vi "MegaAwesome_9_24_12a_JW.vi"() -> ()   [LabVIEW 2011]
uses:
  MegaAwesome_States.ctl
  <vilib>/Utility/inputDevices.llb/keyboardAcquire.vi
  <vilib>/Utility/file.llb/Read From Spreadsheet File (string).vi
  <vilib>/Utility/file.llb/Write To Spreadsheet File (string).vi
panel:
  out "Image Center X":i32
  in  "Disable Flag":bool
  out "Index":string
  out "ROI Descriptor out":T1 {"Contours"."Type" items=["No Selection", "Point", "Line", "Rectangle", "Oval", "Polygon", "Freehand Region", "Annulus", "Unused2", "Unused3", "Broken Line", "Freehand Line", "Rotated Rectangle"]}
  out "ROI Descriptor":T1 {"Contours"."Type" items=["No Selection", "Point", "Line", "Rectangle", "Oval", "Polygon", "Freehand Region", "Annulus", "Unused2", "Unused3", "Broken Line", "Freehand Line", "Rotated Rectangle"]}
  in  "Slider Min":dbl=5.0
  in  "Slider Max":dbl=5.0
  out "Opj X Axis":string
  out "X Axis Display Type":string
  in  "Index-Sat":dbl=5.0
  in  "Index-Lin":dbl=5.0
  in  "IndexLog-Lin":dbl=5.0
  in  "IndexLog-Sat":dbl=5.0 caption="Num Pts"
  out "Lin Id-Log Used":dbl[](array[numeric])
  out "Lin-Vg Array-Log Used":dbl[](array[numeric])
  in  "New: Comments":string
  out "Save Array":string[][](array[string])
  out "Folder Index":i32 caption="Length"
  out "Sat Id-Used":dbl[](array[numeric])
  out "Sat Vg Array-Used":dbl[](array[numeric])
  out "Vg Array-Log-Used":dbl[](array[numeric])
  out "Sat Id-Log-Used":dbl[](array[numeric])
  out "Lin Id-Used":dbl[](array[numeric])
  out "Lin-Vg Array-Used":dbl[](array[numeric])
  out "Lin Vd":dbl
  out "Recorded Prop":T2
  out "Current State":T3
  in  "Main Tab Control":T4(tab)
  in  "OE Link":bool
  in  "Transfer File":path
  out "Transfer Folder":path
  in  "1) Transport":bool caption="2) Transport"
  in  "Image Analysis":bool caption="1) Image Analysis"
  in  "Transport\nFolder":path caption="Transport Folder"
  out "Transport\nFile":path=path "D:/UserData/Desktop/Jeremy/WFU/Research/Programs/VI mods/Image Not Found.png" caption="Transport File"
  in  "Image Folder":path
  out "Image File":path=path "D:/UserData/Desktop/Jeremy/WFU/Research/Programs/VI mods/Image Not Found.png"
  out "Fabrication Prop":T5
  out "Distances":dbl[](array[numeric])
  in  "Zoom":i16(slide)=-3 scale=-5.0..5.0
  in  "Magnification":u16(ring) items=["5x", "10x", "20x", "50x", "80x"]
  in  "Undo Button":bool
  in  "Remove Button":bool
  in  "Transfer Plots":T6(tab)=enum."Saturation"
  in  "Lin-Trans Slider":dbl(slide) step=1.0 scale=-4.0..4.0 scale format="%#_1p"
  out "Sqrt-Lin":cluster{dbl[], dbl[]}[](graph)
  in  "Sat-Trans Slider":dbl(slide) step=1.0 scale=-4.0..4.0 scale format="%#_1p"
  out "Sqrt-Sat":cluster{dbl[], dbl[]}[](graph)
  out "Raw- Lin":cluster{dbl[], dbl[]}[](graph)
  out "Raw- Sat":cluster{dbl[], dbl[]}[](graph)
  in  "Log Plots":enum32{"Linear", "Saturation", "Transport"}(tab)=enum."Saturation"
  in  "Lin-Log Slider":dbl(slide) step=1.0 scale=-4.0..4.0 scale format="%#_1p"
  out "Lin-Log":cluster{dbl[], dbl[]}[](graph)
  in  "Sat-Log Slider":dbl(slide) step=1.0 scale=-4.0..4.0 scale format="%#_1p"
  out "Sat-Log":cluster{dbl[], dbl[]}[](graph)
  out "Transport":cluster{dbl[], dbl[]}[](graph)
  out "Transport Name:":string
  in  "Manual Controls":T7
  in  "File Controls":T8
  out "Date Recorded":string="Date Recorded" caption="Measured"
  out "Data Name:":string
  out "Image Name":string
  out "Date Created":string caption="Fabricated"
  in  "Comments:":string
  out "Rec: Length":dbl caption="Length" format="%#_3g"
  out "Rec: Width":dbl caption="Width" format="%#_4g"
  out "Rec: Dielectric (d)":dbl caption="Dielectric (d)" format="%#_3g"
  in  "New: Dielectric":dbl
  in  "New: Length":dbl
  in  "New: Width":dbl
  out "Rec: Temp":dbl caption="Sample Temp" format="%.1f"
  in  "New: Temp":dbl format="%.1f"
  out "Image Out":T9(plugin-control)
  in  "Num Pts":dbl=5.0
  in  "Num Pts Log":dbl=5.0 caption="Num Pts"
  out "Recorded Values Cluster":T10
  out "Calculated Values Cluster":T10 caption="Recorded Values Cluster"
  out "Re-Calculated Values Cluster":T10 caption="Recorded Values Cluster"
  in  "Independant Variable:":string(combo)="Length (um):"
  out "Image Preview":T9(plugin-control)
  out "Total Width":dbl
  in  "Index Array":u16(ring) caption="Index" items=["1A", "1A", "1A", "1A", "1A", "1A", "1A", "1A", "1A", "1A", "1A", "1A", "1A", "1A", "1A", "1A", "1A", "1A", "1A", "1A", "1A", "1A", "1A", "1A", "1A", "1A", "1A", "1A", "1A", "1A", "1A", "1A", "1A", "1A", "1A", "1A", "1A"]
  in  "Room Temp":dbl=294.0 caption="Room Temp (K)"
  out "No Image\n File":path=path "\\\\acad1\\physics/Jurchescu-group/JW-PD/Mega Awesome/Image Not Found.png" caption="No Image File"
  out "Origin Project File":path=path "\\\\acad1\\physics/Jurchescu-group/JW-PD/Group Library/Origin Project Files/DeviceData_8_10_12a_JW.opj"
  out "No Transport\n File":path=path "\\\\acad1\\physics/Jurchescu-group/JW-PD/Mega Awesome/No Transport File.txt" caption="No Transport File"
  in  "Transport Style Controls":T11={"Transport Line Size"=1, "Transport Line Color"=16772608} {"Transport Line Size" items=["Extra Small", "Small", "Medium", "Large", "Extra Large"]}
  out "Application Directory":path
  # "1)  Select the Transfer File that you would like to analyze:"
  # "Transfer Location"
  # "2) What else would you like to view during your analysis?"
  # "Transport Location"
  # "Image Location"
  # "Recorded"
  # "Calculated"
  # "Re-Calculated"
  # "Manual"
  # "um"
  # "Slider\nDoesn't\nWork"
  # "V"
  # "V"
  # "Slider\nDoesn't\nWork"
  # "V"
  # "Default File Choices"
  # "Default Analysis Values"
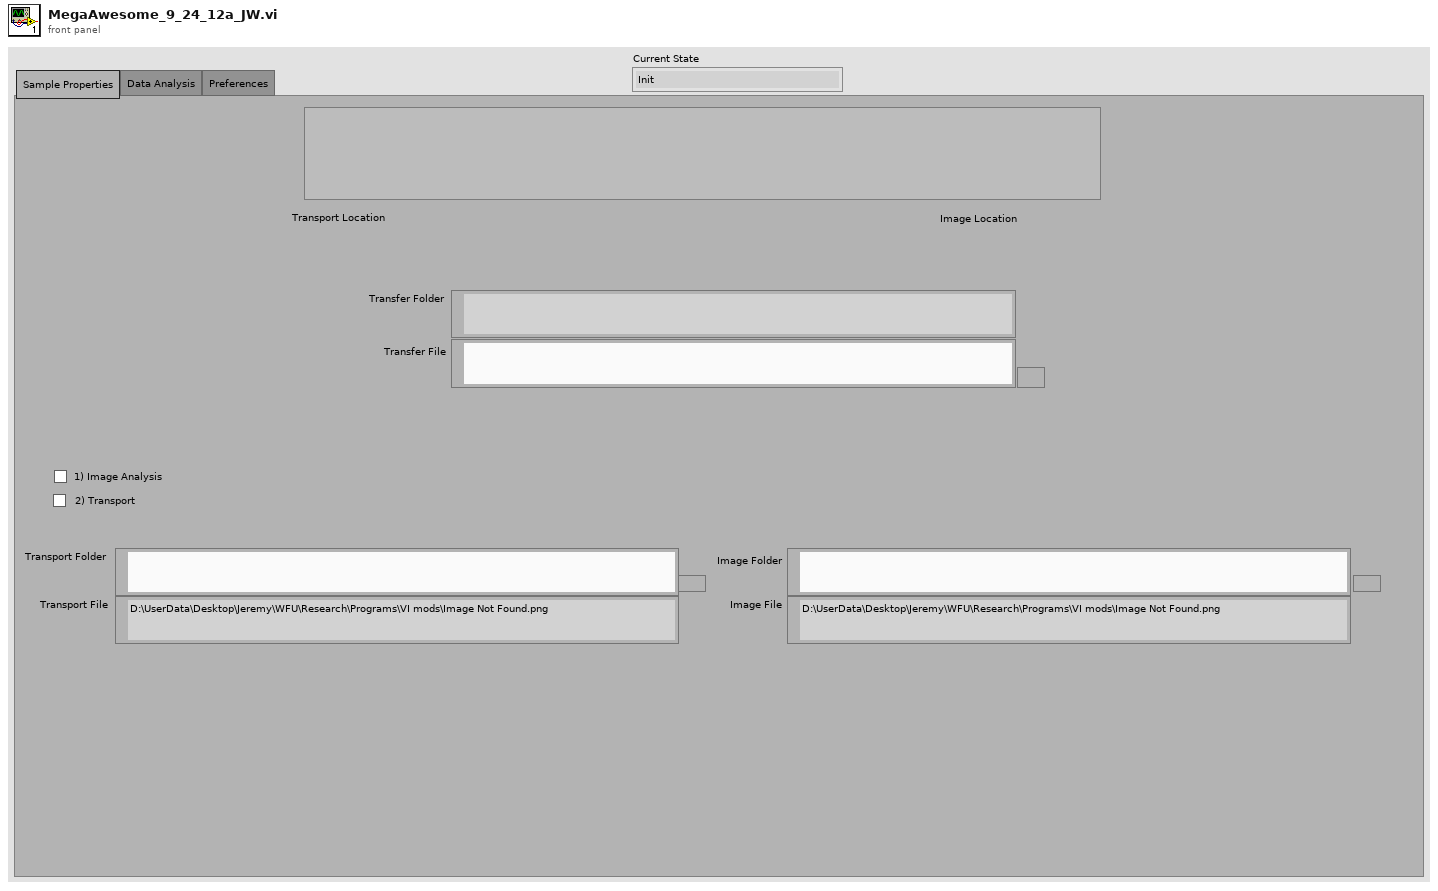
[diagram p1: front panel]
types:
  T1 = typedef "ROI Descriptor" = cluster{"Global Rectangle":i32[], "Contours":cluster{"ID":enum32{"External", "Internal"}, "Type":u32, "Coordinates":i32[]}[]}
  T2 = cluster{"Date Recorded":string, "Index":string, "Length":dbl, "Width":dbl, "Sample Temp":dbl}
  T3 = typedef "MegaAwesome_States.ctl" = enum16{"Init", "File Missing", "No Event", "Read Data", "Calculated Values", "Re-Calculated Values", "Next File", "Previous File", "Discard File", "Save", "Save Lines", "Export", "Exit"}
  T4 = enum32{"Sample Properties", "Data Analysis", "Preferences"}
  T5 = cluster{"Date Created":string, "Material":string, "Solvent":string, "Concentration":dbl, "Method":string, "Dielectric (nm)":dbl, "Treatment":string, "Comments":string}
  T6 = enum32{"Linear", "Saturation", "Raw-Linear", "Raw-Saturation"}
  T7 = cluster{"Manual-Temp":bool, "Manual-Width":bool, "Manuel-Length":bool, "Manuel-Dielectric":bool, "Manual Comments":bool}
  T8 = cluster{"Previous File":bool, "Discard ":bool, "Save Lines":bool, "Close":bool, "Next File ":bool, "Save":bool, "Save Next":bool, "Export":bool}
  T9 = typedef "IMAQ Image.ctl" = refnum<image>
  T10 = cluster{"Mobility-Sat":dbl, "Moblitity-Lin":dbl, "On/Off":dbl, "Off Current":dbl, "Vt-Sat":dbl, "STS":dbl, "Trap Density-VT":dbl, "Trap Density-STS":dbl}
  T11 = cluster{"Transport Line Size":u16, "Transport Line Color":u32}
  T12 = typedef "LVBoundsTypeDef.ctl" = cluster{"Width":u32, "Height":u32}
  T13 = cluster{"Global Rectangle":i32[], "Contours":cluster{"Contour Type":u32, "ROI Type":u32, "Points":i32[]}[]}
  T14 = cluster{"Contour Type":u32, "ROI Type":u32, "Points":i32[]}[]
  T15 = cluster{i32[], cluster{"Contour Type":u32, "ROI Type":u32, "Points":i32[]}[]}
  T16 = enum16{"0", "1", "2", "3", "4", "5", "6", "7", "8", "9", "A", "B", "C", "D", "E", "F", "G", "H", "I", "J", "K", "L", "M", "N", "O", "P", "Q", "R", "S", "T", "U", "V", "W", "X", "Y", "Z", "F1", "F2", "F3", "F4", "F5", "F6", "F7", "F8", "F9", "F10", "F11", "F12", "F13", "F14", "F15", "ADD", "BACK", "BACKSLASH", "CAPITAL", "COMMA", "DECIMAL", "DELETE", "DIVIDE", "DOWN", "END", "EQUALS", "ESCAPE", "GRAVE (`)", "HOME", "INSERT", "LBRACKET", "LCONTROL", "LEFT", "L ALT", "LSHIFT", "LWIN", "MINUS", "MULTIPLY", "NEXT", "NUMLOCK", "NUMPAD_0", "NUMPAD_1", "NUMPAD_2", "NUMPAD_3", "NUMPAD_4", "NUMPAD_5", "NUMPAD_6", "NUMPAD_7", "NUMPAD_8", "NUMPAD_9", "PAUSE", "PERIOD", "PRIOR (PG UP)", "RBRACKET", "RCONTROL", "RETURN", "RIGHT", "R ALT", "RSHIFT", "RWIN", "SCROLL", "SEMICOLON", "SLASH", "SPACE", "SUBTRACT", "TAB", "UP", "ENTER (num pad)", "' (quote)"}[]
  T17 = enum16{"0", "1", "2", "3", "4", "5", "6", "7", "8", "9", "A", "B", "C", "D", "E", "F", "G", "H", "I", "J", "K", "L", "M", "N", "O", "P", "Q", "R", "S", "T", "U", "V", "W", "X", "Y", "Z", "F1", "F2", "F3", "F4", "F5", "F6", "F7", "F8", "F9", "F10", "F11", "F12", "F13", "F14", "F15", "ADD", "BACK", "BACKSLASH", "CAPITAL", "COMMA", "DECIMAL", "DELETE", "DIVIDE", "DOWN", "END", "EQUALS", "ESCAPE", "GRAVE (`)", "HOME", "INSERT", "LBRACKET", "LCONTROL", "LEFT", "L ALT", "LSHIFT", "LWIN", "MINUS", "MULTIPLY", "NEXT", "NUMLOCK", "NUMPAD_0", "NUMPAD_1", "NUMPAD_2", "NUMPAD_3", "NUMPAD_4", "NUMPAD_5", "NUMPAD_6", "NUMPAD_7", "NUMPAD_8", "NUMPAD_9", "PAUSE", "PERIOD", "PRIOR (PG UP)", "RBRACKET", "RCONTROL", "RETURN", "RIGHT", "R ALT", "RSHIFT", "RWIN", "SCROLL", "SEMICOLON", "SLASH", "SPACE", "SUBTRACT", "TAB", "UP", "ENTER (num pad)", "' (quote)"}
  T18 = cluster{string, sgl, bool, bool, bool, bool, bool, bool, i32}
  T19 = cluster{i32, cluster{string, sgl, bool, bool, bool, bool, bool, bool, i32}, i32, i32}
  T20 = cluster{"Contour Type":u32, "ROI Type":u32, "Points":i32[]}
  T21 = cluster{"Points[0]":i32, "Points[1]":i32, "Points[2]":i32, "Points[3]":i32, "Points[4]":i32, "Points[5]":i32, "Points[6]":i32, "Points[7]":i32, "Points[8]":i32}
  T22 = cluster{"[0]":cluster{dbl[], dbl[]}, "[1]":cluster{dbl[], dbl[]}, "[2]":cluster{dbl[], dbl[]}, "[3]":cluster{dbl[], dbl[]}, "[4]":cluster{dbl[], dbl[]}, "[5]":cluster{dbl[], dbl[]}, "[6]":cluster{dbl[], dbl[]}, "[7]":cluster{dbl[], dbl[]}, "[8]":cluster{dbl[], dbl[]}}
  T23 = cluster{"Sat Vg Used":dbl[], "Sat Sqrt(Id) Used ":dbl[], "Lin Vg Used":dbl[], "Lin Sqrt(Id) Used":dbl[], "Index-Lin":dbl, "Index-Sat":dbl}
  T24 = cluster{"Raw Sat":cluster{dbl[], dbl[]}[], "Sqrt Sat":cluster{dbl[], dbl[]}[], "Log Sat":cluster{dbl[], dbl[]}[], "Raw Lin":cluster{dbl[], dbl[]}[], "Sqrt Lin":cluster{dbl[], dbl[]}[], "Log Lin":cluster{dbl[], dbl[]}[]}
  T25 = cluster{"Mobility-Sat":dbl, "Vt-Sat":dbl, "Mobility-Lin":dbl, "Vt-Lin":dbl, "Off I-Sat":dbl, "On/Off I-Sat":dbl}
  T26 = cluster{"Sat Vg Used":dbl[], "Sat Log(Id) Used":dbl[], "Lin Vg Used":dbl[], "Lin Log(Id) Used":dbl[], "STS Index-Sat":dbl, "STS Index-Lin":dbl}
  T27 = cluster{"Independant  Variable Indicator":string, "Parameter String Indicator":string}
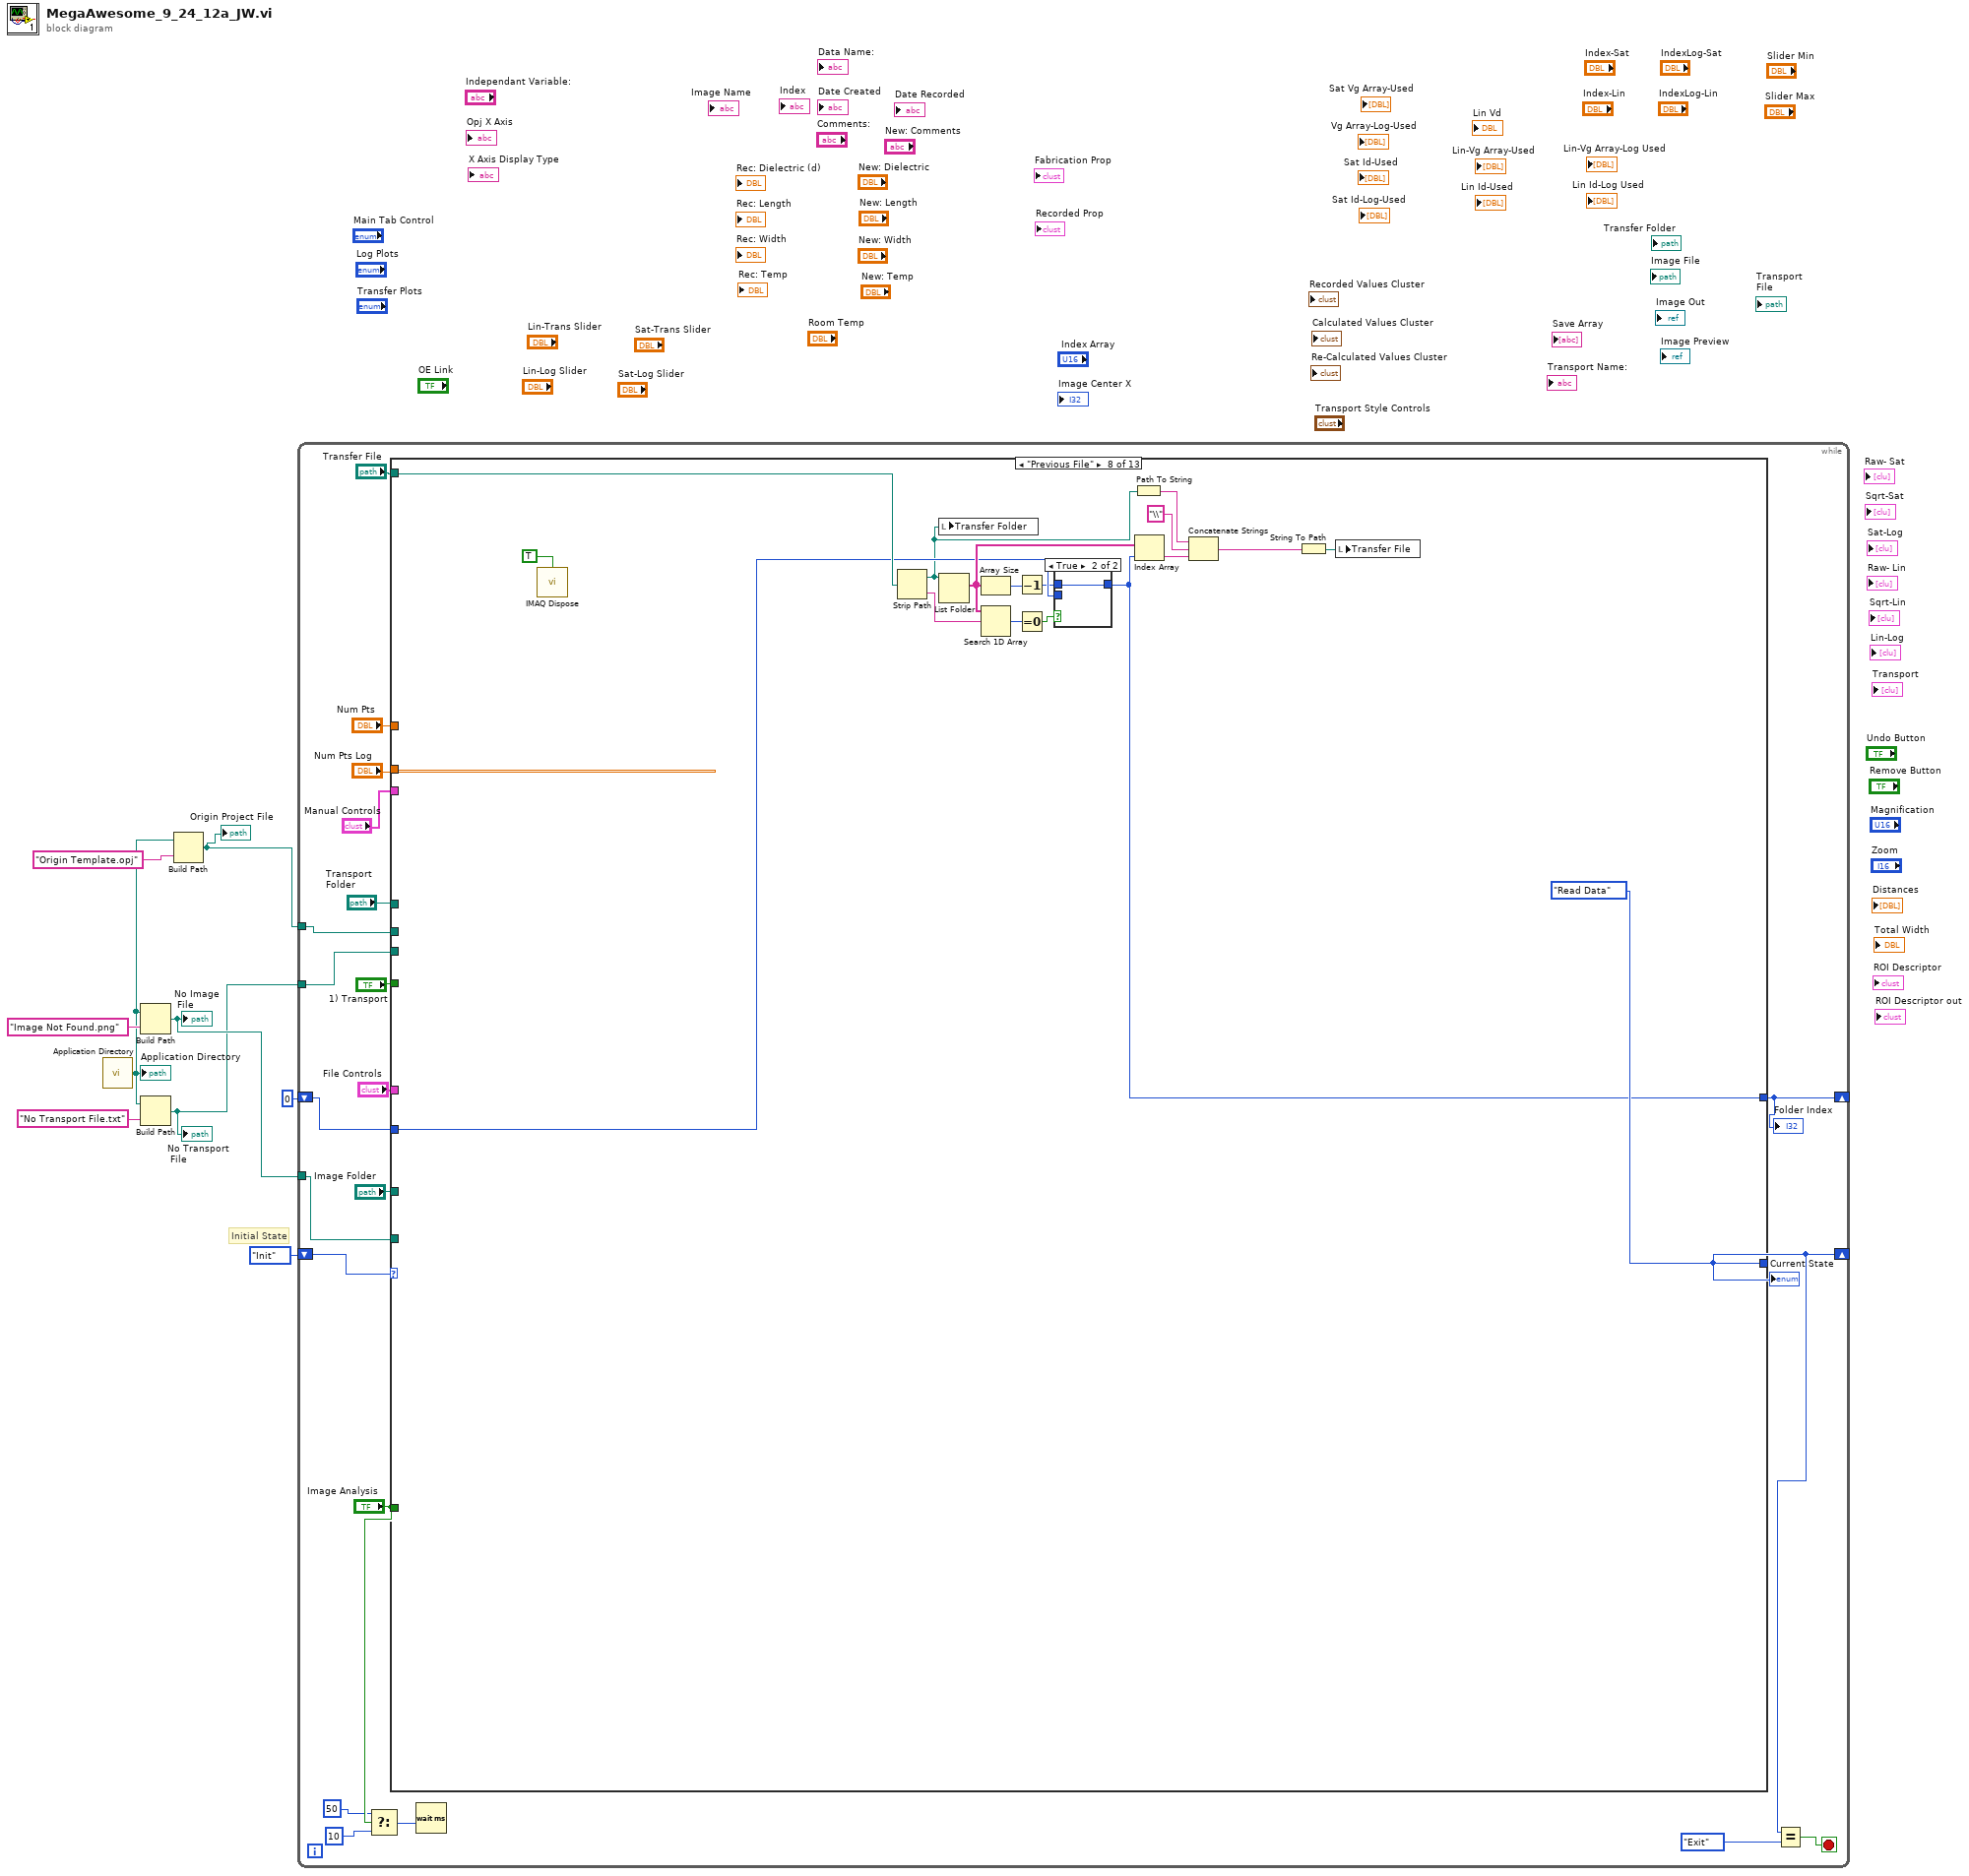
[diagram p0: block diagram]
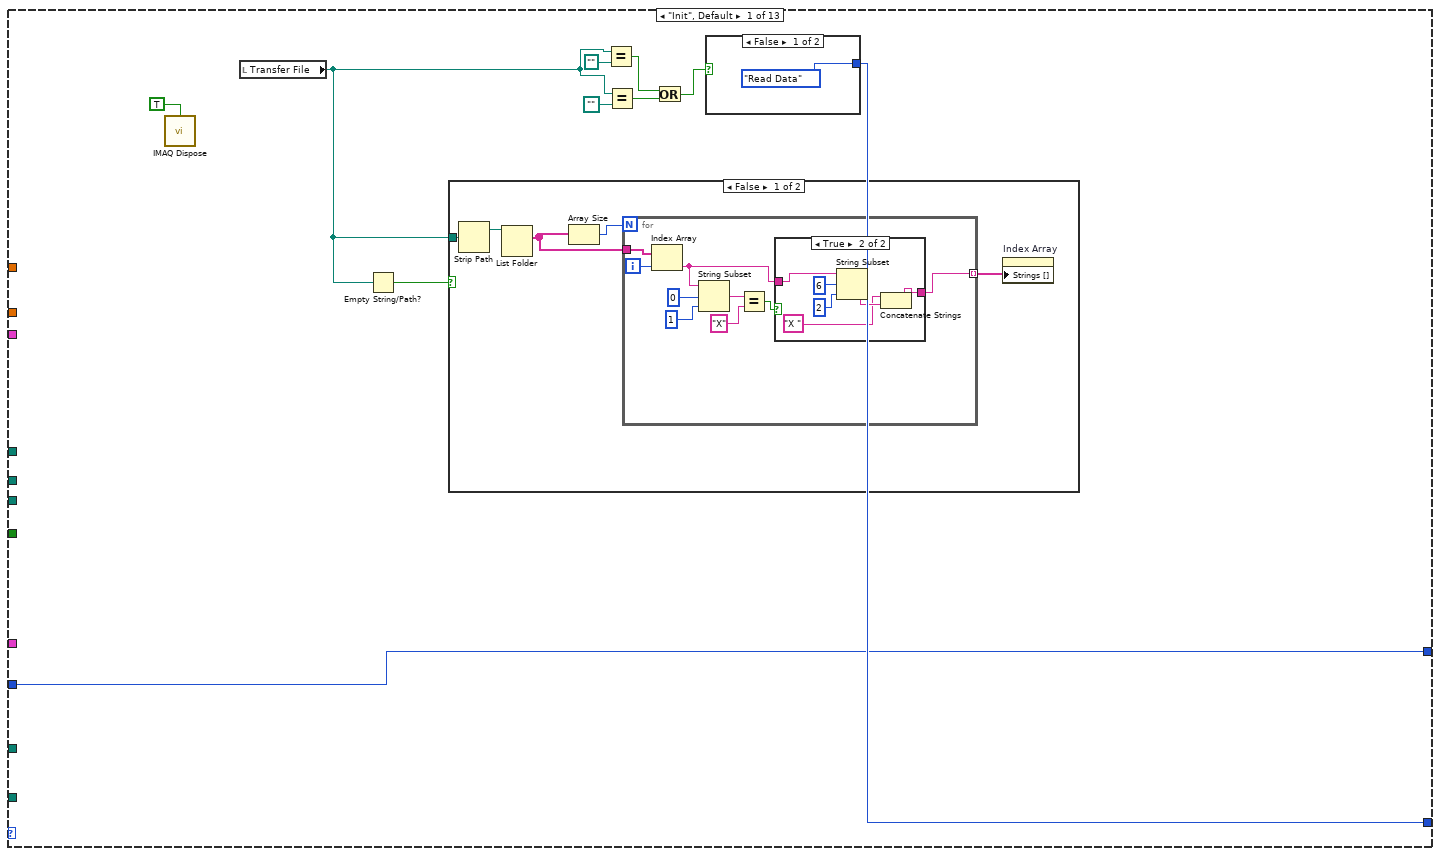
[diagram p2: hidden frame]
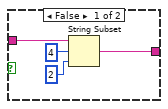
[diagram p3: hidden frame]
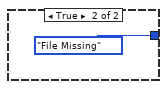
[diagram p5: hidden frame]
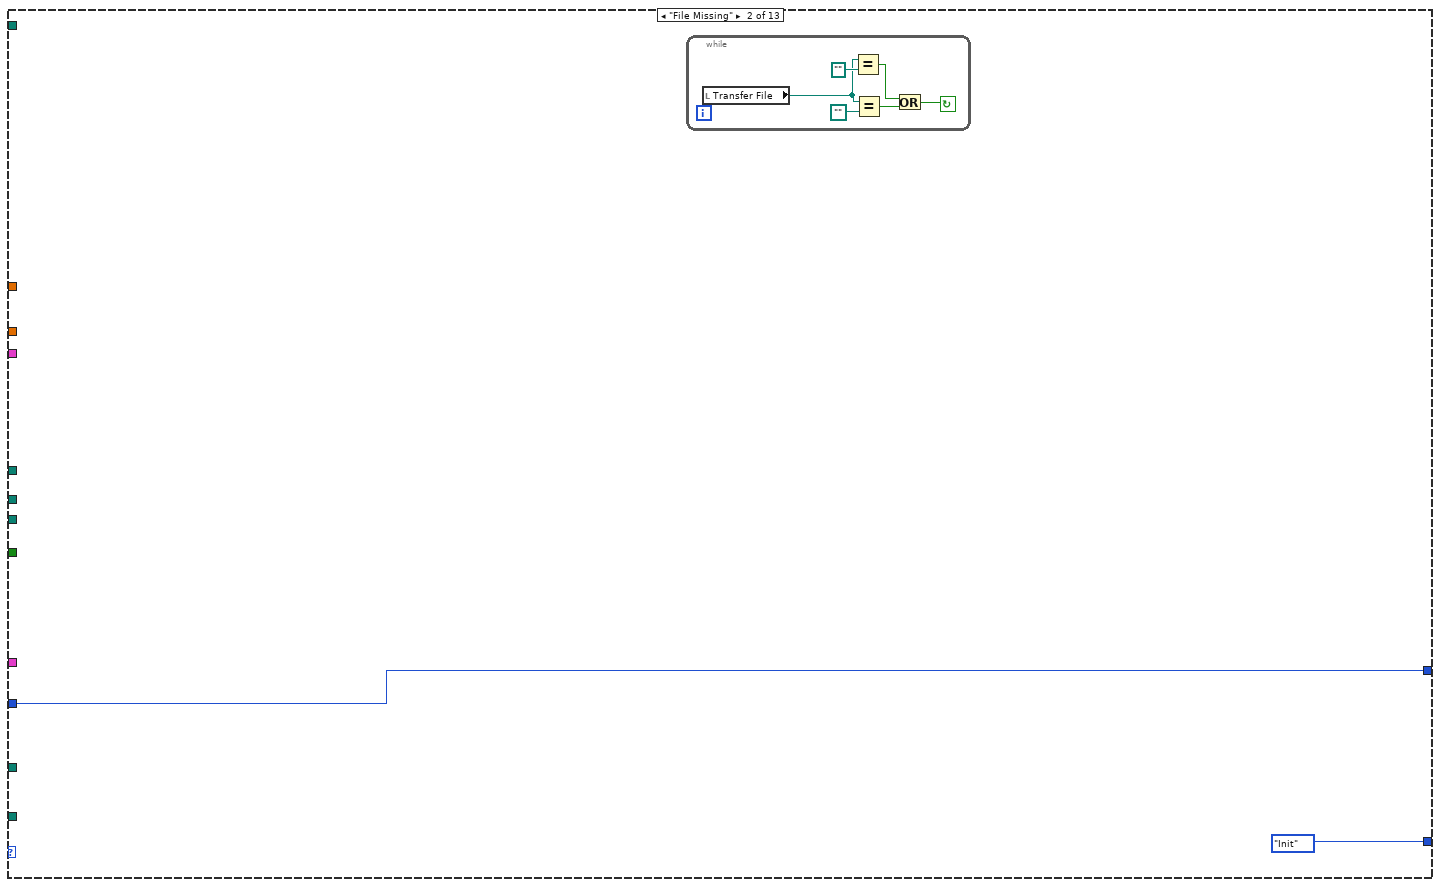
[diagram p6: hidden frame]
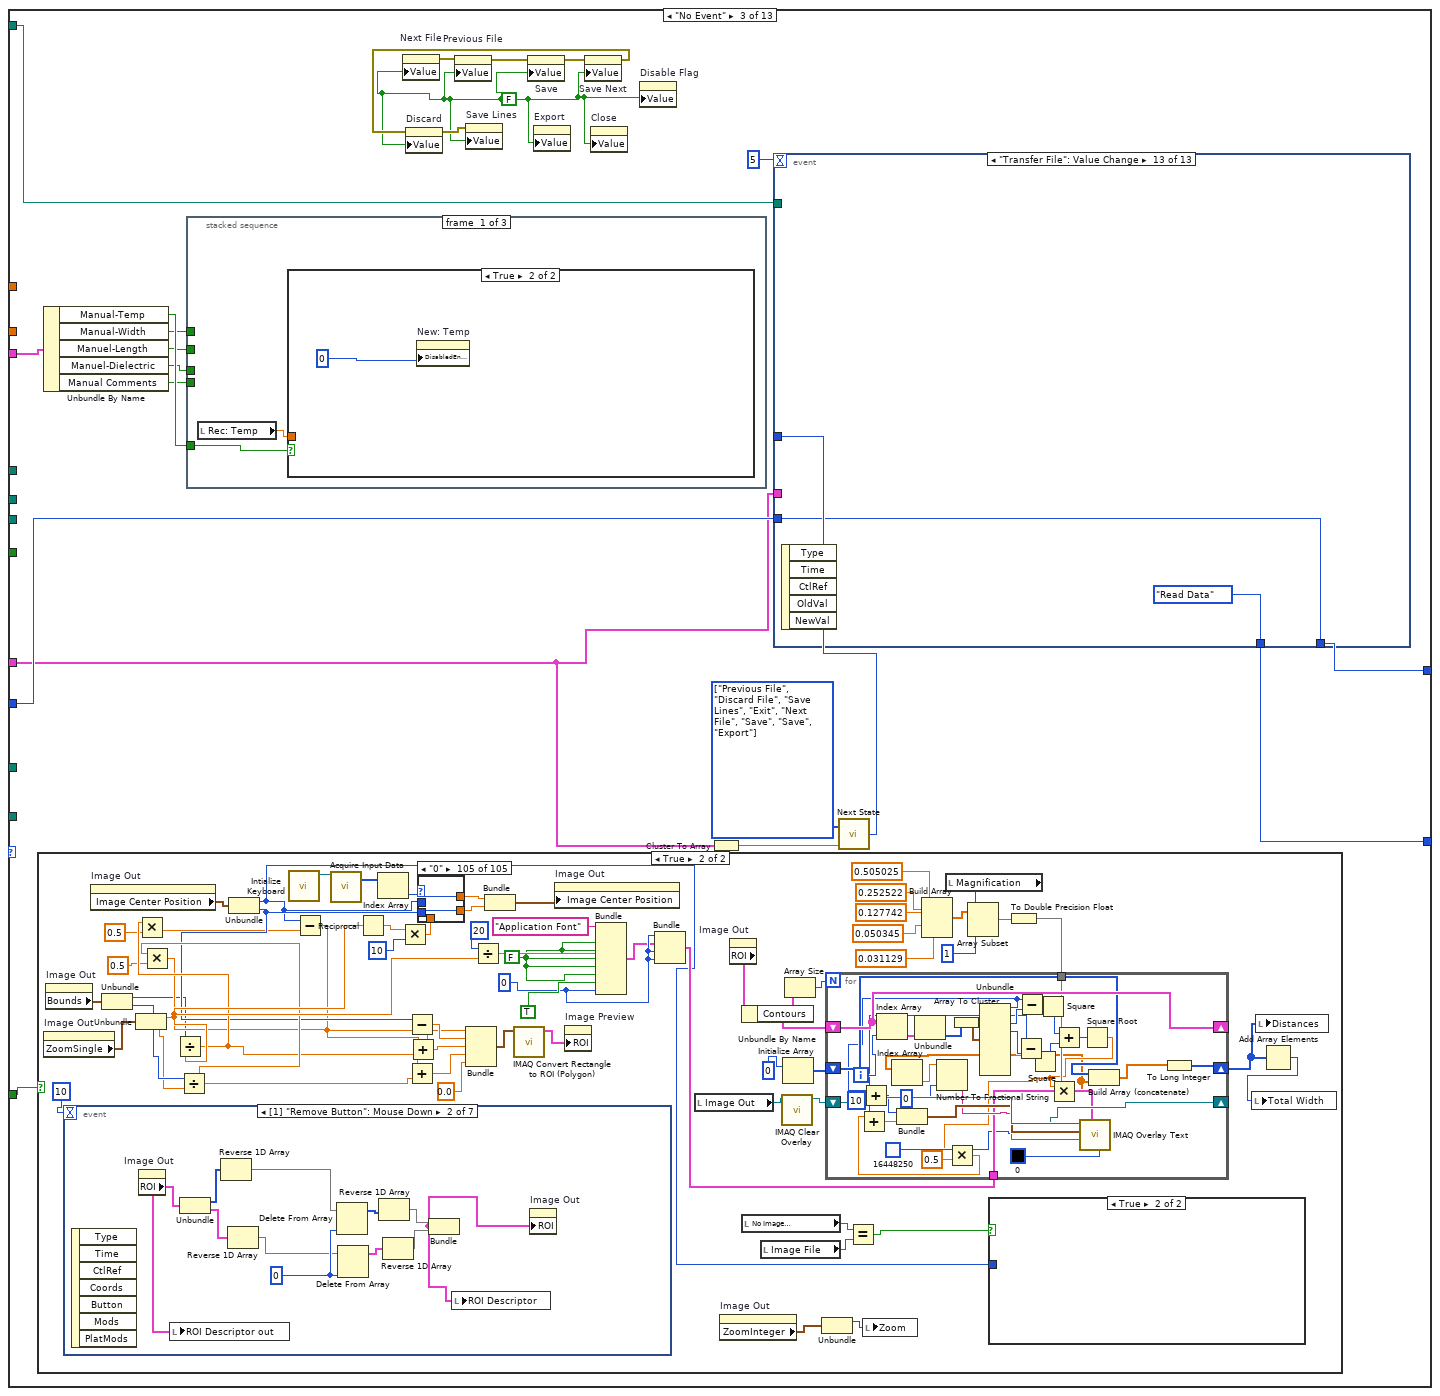
[diagram p7: hidden frame]
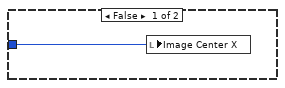
[diagram p9: hidden frame]
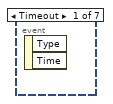
[diagram p10: hidden frame]
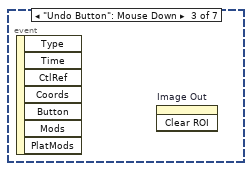
[diagram p11: hidden frame]
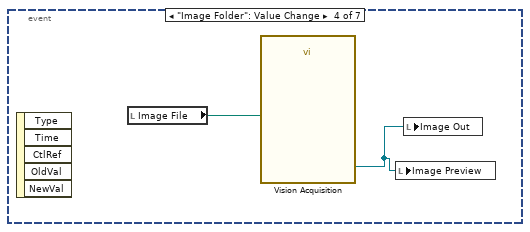
[diagram p12: hidden frame]
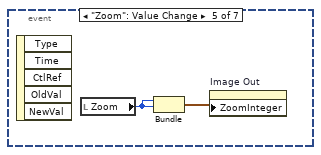
[diagram p13: hidden frame]
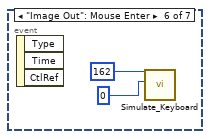
[diagram p14: hidden frame]
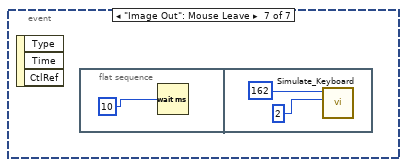
[diagram p15: hidden frame]
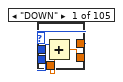
[diagram p16: hidden frame]
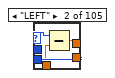
[diagram p17: hidden frame]
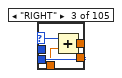
[diagram p18: hidden frame]
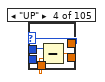
[diagram p19: hidden frame]
diagram:
  # "Initial State"
  n1 = call <vilib>:"Application Directory.vi"() -> ("Application Directory"=w2:path)
  "Application Directory" <- w2
  n2 = Build Path(base path=w2, name or relative path="Image Not Found.png") -> (appended path=w5:path)
  "No Image\n File" <- w5
  n3 = Build Path(base path=w2, name or relative path="No Transport File.txt") -> (appended path=w4:path)
  "No Transport\n File" <- w4
  n4 = Build Path(base path=w2, name or relative path="Origin Template.opj") -> (appended path=w3:path)
  "Origin Project File" <- w3
  n5 = while {
    shift-right: [w10] -> _
    shift-left: MegaAwesome_States."Init" -> [w29]
    shift-right: [w22] -> _
    shift-left: 0 -> [w23]
    tunnel: w5 -> [w14]
    tunnel: w4 -> [w12]
    tunnel: w3 -> [w11]
    stop <- w30 stop-if-true
    n6 = Select(t=50, s="Image Analysis", f=10) -> (s? t:f=w16:i32)
    n7 = case shown="\"Previous File\"" w29 {
      tunnel: [w35 MegaAwesome_States."Init" w87 MegaAwesome_States."Calculated Values" MegaAwesome_States."Re-Calculated Values" MegaAwesome_States."No Event" MegaAwesome_States."Read Data" MegaAwesome_States."Read Data" MegaAwesome_States."Init" w822 MegaAwesome_States."Exit" MegaAwesome_States."No Event" MegaAwesome_States."Exit"] -> w10
      tunnel: "Transfer File" -> [_ _ w77 w595 w642 _ w763 w774 w792 w827 _ _ _]
      tunnel: "Num Pts" -> [_ _ _ _ w666 _ _ _ _ _ _ _ _]
      tunnel: "Num Pts Log" -> [_ _ _ _ w665 _ _ _ _ _ _ _ _]
      tunnel: "Image Folder" -> [_ _ _ _ w662 _ _ _ _ _ _ w1346 _]
      tunnel: w14 -> [_ _ _ _ w661 _ _ _ _ _ _ _ _]
      tunnel: [w34 w67 w78 w600 w660 w723 w749 w772 w787 w828 w1344 w1356 w1361] -> w22
      tunnel: w23 -> [w34 w67 w79 w598 w660 w723 w750 w773 _ w828 w1344 w1356 w1361]
      tunnel: "Manual Controls" -> [_ _ w89 _ _ _ _ _ _ w826 _ _ _]
      tunnel: "File Controls" -> [_ _ w75 _ _ _ _ _ _ w821 _ _ _]
      tunnel: "1) Transport" -> [_ _ _ _ w633 _ _ _ _ _ _ _ _]
      tunnel: "Image Analysis" -> [_ _ w80 _ w632 _ _ _ _ _ _ _ _]
      tunnel: "Transport\nFolder" -> [_ _ _ _ w631 _ _ _ _ _ _ _ _]
      tunnel: w12 -> [_ _ _ _ w630 _ _ _ _ _ _ _ _]
      tunnel: w11 -> [_ _ _ _ _ _ _ _ _ _ _ _ w1360]
      frame "Init", Default {
        n8 = call "IMAQ Dispose"("All Images? (No)"=TRUE) -> ()  [unwired: 5 in, 1 out]
        n9 = local read "Transfer File"() -> (w32:path)
        n10 = Empty String/Path?(string/path=w32) -> (empty?=w33:bool)
        n11 = case shown="False" w33 {
          tunnel: w32 -> [w42 _]
          frame False {
            n12 = Strip Path(path=w42) -> (stripped path=w44:path)  [unwired: 1 out]
            n13 = List Folder(path=w44) -> (filenames=w43:string[])  [unwired: 3 in, 3 out]
            n14 = Array Size(array=w43) -> (size(s)=w45:i32)
            n15 = for {
              N: w45 -> [_]
              tunnel: w43 -> [w54]
              tunnel: [w52] -> w41 mode=indexing
              i -> [w53]
              n16 = Index Array(array=w54, index=w53) -> (element=w51:string)
              n17 = String Subset(string=w51, offset (0)=0, length (rest)=1) -> (substring=w48:string)
              n18 = Equal?(x=w48, y="X") -> (x = y?=w47:bool)
              n19 = case shown="True" w47 {
                tunnel: w51 -> [w58 w62]
                tunnel: [w55 w61] -> w52
                frame False {
                  n20 = String Subset(string=w58, offset (0)=4, length (rest)=2) -> (substring=w55:string)
                }
                frame True {
                  n21 = String Subset(string=w62, offset (0)=6, length (rest)=2) -> (substring=w60:string)
                  n22 = Concatenate Strings("X ", w60) -> (w61:string)
                }
              }
            }
            n23 = property on="Index Array" class="Ring (strict)"("Strings []"=w41) -> ()  [unwired: 2 in, 2 out]
          }
          frame True {
          }
        }
        n24 = Equal?(x=w32, y=path "") -> (x = y?=w38:bool)
        n25 = Equal?(x=w32, y=path "") -> (x = y?=w37:bool)
        n26 = Or(x=w38, y=w37) -> (x .or. y?=w40:bool)
        n27 = case shown="False" w40 {
          tunnel: [MegaAwesome_States."Read Data" MegaAwesome_States."File Missing"] -> w35
          frame False {
          }
          frame True {
          }
        }
      }
      frame "File Missing" {
        n28 = while {
          stop <- w69 continue-if-true
          n29 = local read "Transfer File"() -> (w70:path)
          n30 = Equal?(x=w70, y=path "") -> (x = y?=w72:bool)
          n31 = Equal?(x=w70, y=path "") -> (x = y?=w73:bool)
          n32 = Or(x=w72, y=w73) -> (x .or. y?=w69:bool)
        }
      }
      frame "No Event" {
        w76 = FALSE
        w96 = T3[] [enum."Previous File", enum."Discard File", enum."Save Lines", enum."Exit", enum."Next File", enum."Save", enum."Save", enum."Export"] items=["Init", "File Missing", "No Event", "Read Data", "Calculated Values", "Re-Calculated Values", "Next File", "Previous File", "Discard File", "Save", "Save Lines", "Export", "Exit"]
        n33 = case shown="True" w80 {
          frame False {
          }
          frame True {
            w152 = FALSE
            w154 = 0
            n34 = property on="Image Out" class="ImageControl"() -> ("ZoomSingle"=w138:cluster{"X":sgl, "Y":sgl})  [unwired: 2 in, 2 out]
            n35 = property on="Image Out" class="ImageControl"() -> ("Bounds"=w137:T12)  [unwired: 2 in, 2 out]
            n36 = event shown="[1] \"Remove Button\": Mouse Down" {
              selector: _ -> [_ _ _ _ _ _ _]
              dyn-events: _ -> [_ _ _ _ _ _ _]
              timeout: 10 -> [_ _ _ _ _ _ _]
              event Timeout {
                n37 = event-data() -> ()  [unwired: 1 in, 2 out]
              }
              event "Remove Button": Mouse Down {
                w172 = 0
                n38 = event-data() -> ()  [unwired: 1 in, 7 out]
                n39 = property on="Image Out" class="ImageControl"() -> ("ROI"=w162:T13)  [unwired: 2 in, 2 out]
                n40 = local write "ROI Descriptor out"(w162) -> ()
                n41 = Unbundle(w162) -> ("Global Rectangle"=w171:i32[], "Contours"=w169:T14)
                n42 = Reverse 1D Array(array=w171) -> (reversed array=w170:i32[])
                n43 = Reverse 1D Array(array=w169) -> (reversed array=w168:T14)
                n44 = Delete From Array(array=w170, index=w172) -> (array with subset deleted=w167:i32[])  [unwired: 1 in, 1 out]
                n45 = Delete From Array(array=w168, index=w172) -> (array with subset deleted=w166:T14)  [unwired: 1 in, 1 out]
                n46 = Reverse 1D Array(array=w167) -> (reversed array=w165:i32[])
                n47 = Reverse 1D Array(array=w166) -> (reversed array=w164:T14)
                n48 = Bundle(w165, w164) -> (w163:T15)  [unwired: 1 in]
                n49 = local write "ROI Descriptor"(w163) -> ()
                n50 = property on="Image Out" class="ImageControl"("ROI"=w163) -> ()  [unwired: 2 in, 2 out]
              }
              event "Undo Button": Mouse Down {
                n51 = event-data() -> ()  [unwired: 1 in, 7 out]
                n52 = invoke on="Image Out" class="ImageControl" method="Clear ROI"() -> ()  [unwired: 3 in, 3 out]
              }
              event "Image Folder": Value Change {
                n53 = event-data() -> ()  [unwired: 1 in, 5 out]
                n54 = local read "Image File"() -> (w174:path)
                n55 = call "Vision Acquisition"("Image Path"=w174) -> ("Image Out"=w173:T9)  [unwired: 25 in, 1 out]
                n56 = local write "Image Preview"(w173) -> ()
                n57 = local write "Image Out"(w173) -> ()
              }
              event "Zoom": Value Change {
                n58 = event-data() -> ()  [unwired: 1 in, 5 out]
                n59 = local read "Zoom"() -> (w175:i16)
                n60 = Bundle("Zoom"=w175, "Zoom"=w175) -> (w176:cluster{"Zoom":i16, "Zoom":i16})  [unwired: 1 in]
                n61 = property on="Image Out" class="ImageControl"("ZoomInteger"=w176) -> ()  [unwired: 2 in, 2 out]
              }
              event "Image Out": Mouse Enter {
                n62 = event-data() -> ()  [unwired: 1 in, 3 out]
                n63 = call "Simulate_Keyboard.vi"("Action"=0, "Virtual Key"=162) -> ()  [unwired: 7 in, 1 out]
              }
              event "Image Out": Mouse Leave {
                n64 = event-data() -> ()  [unwired: 1 in, 3 out]
                n65 = flat-sequence {
                  frame #0 {
                    n66 = Wait (ms)(milliseconds to wait=10) -> ()  [unwired: 1 out]
                  }
                  frame #1 {
                    n67 = call "Simulate_Keyboard.vi"("Action"=2, "Virtual Key"=162) -> ()  [unwired: 7 in, 1 out]
                  }
                }
              }
            }
            n68 = property on="Image Out" class="ImageControl"() -> ("Image Center Position"=w131:cluster{"X":u32, "Y":u32})  [unwired: 2 in, 2 out]
            n69 = Unbundle(w137) -> ("Width"=w140:u32, "Height"=w141:u32)
            n70 = Unbundle(w138) -> ("X"=w158:sgl, "Y"=w139:sgl)
            n71 = Divide(x=w140, y=w158) -> (x/y=w149:sgl)
            n72 = Multiply(x=w149, y=0.5) -> (x*y=w144:dbl)
            n73 = Divide(x=w141, y=w139) -> (x/y=w150:sgl)
            n74 = Multiply(x=w150, y=0.5) -> (x*y=w145:dbl)
            n75 = Unbundle(w131) -> ("X"=w100:u32, "Y"=w148:u32)
            n76 = call <vilib>:"Intialize Keyboard.vi"() -> ("device ID"=w128:refnum<k1>)  [unwired: 10 in, 1 out]
            n77 = Subtract(x=w100, y=w144) -> (x-y=w146:dbl)
            n78 = call-poly <vilib>:"Acquire Input Data.vi"("device ID"=w128) -> ("keys pressed"=w129:T16)  [unwired: 16 in, 2 out]
            n79 = Reciprocal(x=w158) -> (1/x=w159:sgl)
            n80 = Index Array(array=w129) -> (element=w125:T17)  [unwired: 1 in]
            n81 = Multiply(x=w159, y=10) -> (x*y=w157:sgl)
            n82 = Subtract(x=w148, y=w145) -> (x-y=w147:dbl)
            n83 = Add(x=w147, y=w150) -> (x+y=w133:dbl)
            n84 = Add(x=w146, y=w149) -> (x+y=w132:dbl)
            n85 = case shown="\"0\"" w125 {
              tunnel: w100 -> [w217 w223 w227 w229 w233 w235 w237 w239 w241 w243 w245 w247 w249 w251 w253 w255 w257 w259 w261 w263 w265 w267 w269 w271 w273 w275 w277 w279 w281 w283 w285 w287 w289 w291 w293 w295 w297 w299 w301 w303 w305 w307 w309 w311 w313 w315 w317 w319 w321 w323 w325 w327 w329 w331 w333 w335 w337 w339 w341 w343 w345 w347 w349 w351 w353 w355 w357 w359 w361 w363 w365 w367 w369 w371 w373 w375 w377 w379 w381 w383 w385 w387 w389 w391 w393 w395 w397 w399 w401 w403 w405 w407 w409 w411 w413 w415 w417 w419 w421 w423 w425 w427 w429 w431 w433]
              tunnel: [w217 w222 w226 w229 w233 w235 w237 w239 w241 w243 w245 w247 w249 w251 w253 w255 w257 w259 w261 w263 w265 w267 w269 w271 w273 w275 w277 w279 w281 w283 w285 w287 w289 w291 w293 w295 w297 w299 w301 w303 w305 w307 w309 w311 w313 w315 w317 w319 w321 w323 w325 w327 w329 w331 w333 w335 w337 w339 w341 w343 w345 w347 w349 w351 w353 w355 w357 w359 w361 w363 w365 w367 w369 w371 w373 w375 w377 w379 w381 w383 w385 w387 w389 w391 w393 w395 w397 w399 w401 w403 w405 w407 w409 w411 w413 w415 w417 w419 w421 w423 w425 w427 w429 w431 w433] -> w126
              tunnel: w148 -> [w219 w221 w225 w231 w232 w234 w236 w238 w240 w242 w244 w246 w248 w250 w252 w254 w256 w258 w260 w262 w264 w266 w268 w270 w272 w274 w276 w278 w280 w282 w284 w286 w288 w290 w292 w294 w296 w298 w300 w302 w304 w306 w308 w310 w312 w314 w316 w318 w320 w322 w324 w326 w328 w330 w332 w334 w336 w338 w340 w342 w344 w346 w348 w350 w352 w354 w356 w358 w360 w362 w364 w366 w368 w370 w372 w374 w376 w378 w380 w382 w384 w386 w388 w390 w392 w394 w396 w398 w400 w402 w404 w406 w408 w410 w412 w414 w416 w418 w420 w422 w424 w426 w428 w430 w432]
              tunnel: [w218 w221 w225 w230 w232 w234 w236 w238 w240 w242 w244 w246 w248 w250 w252 w254 w256 w258 w260 w262 w264 w266 w268 w270 w272 w274 w276 w278 w280 w282 w284 w286 w288 w290 w292 w294 w296 w298 w300 w302 w304 w306 w308 w310 w312 w314 w316 w318 w320 w322 w324 w326 w328 w330 w332 w334 w336 w338 w340 w342 w344 w346 w348 w350 w352 w354 w356 w358 w360 w362 w364 w366 w368 w370 w372 w374 w376 w378 w380 w382 w384 w386 w388 w390 w392 w394 w396 w398 w400 w402 w404 w406 w408 w410 w412 w414 w416 w418 w420 w422 w424 w426 w428 w430 w432] -> w127
              tunnel: w157 -> [w216 w220 w224 w228 _ _ _ _ _ _ _ _ _ _ _ _ _ _ _ _ _ _ _ _ _ _ _ _ _ _ _ _ _ _ _ _ _ _ _ _ _ _ _ _ _ _ _ _ _ _ _ _ _ _ _ _ _ _ _ _ _ _ _ _ _ _ _ _ _ _ _ _ _ _ _ _ _ _ _ _ _ _ _ _ _ _ _ _ _ _ _ _ _ _ _ _ _ _ _ _ _ _ _ _ _]
              frame "DOWN" {
                n86 = Add(x=w219, y=w216) -> (x+y=w218:sgl)
              }
              frame "LEFT" {
                n87 = Subtract(x=w223, y=w220) -> (x-y=w222:sgl)
              }
              frame "RIGHT" {
                n88 = Add(x=w227, y=w224) -> (x+y=w226:sgl)
              }
              frame "UP" {
                n89 = Subtract(x=w231, y=w228) -> (x-y=w230:sgl)
              }
              frame "ENTER (num pad)" {
              }
              frame "' (quote)" {
              }
              frame "END" {
              }
              frame "EQUALS" {
              }
              frame "ESCAPE" {
              }
              frame "GRAVE (`)" {
              }
              frame "HOME" {
              }
              frame "INSERT" {
              }
              frame "LBRACKET" {
              }
              frame "LCONTROL" {
              }
              frame "L ALT" {
              }
              frame "LSHIFT" {
              }
              frame "LWIN" {
              }
              frame "MINUS" {
              }
              frame "MULTIPLY" {
              }
              frame "NEXT" {
              }
              frame "NUMLOCK" {
              }
              frame "NUMPAD_0" {
              }
              frame "NUMPAD_1" {
              }
              frame "NUMPAD_2" {
              }
              frame "NUMPAD_3" {
              }
              frame "NUMPAD_4" {
              }
              frame "NUMPAD_5" {
              }
              frame "NUMPAD_6" {
              }
              frame "NUMPAD_7" {
              }
              frame "NUMPAD_8" {
              }
              frame "NUMPAD_9" {
              }
              frame "PAUSE" {
              }
              frame "PERIOD" {
              }
              frame "PRIOR (PG UP)" {
              }
              frame "RBRACKET" {
              }
              frame "RCONTROL" {
              }
              frame "RETURN" {
              }
              frame "R ALT" {
              }
              frame "RSHIFT" {
              }
              frame "RWIN" {
              }
              frame "SCROLL" {
              }
              frame "SEMICOLON" {
              }
              frame "SLASH" {
              }
              frame "SPACE" {
              }
              frame "SUBTRACT" {
              }
              frame "TAB" {
              }
              frame "DIVIDE" {
              }
              frame "DELETE" {
              }
              frame "DECIMAL" {
              }
              frame "COMMA" {
              }
              frame "CAPITAL" {
              }
              frame "BACKSLASH" {
              }
              frame "BACK" {
              }
              frame "ADD" {
              }
              frame "F15" {
              }
              frame "F14" {
              }
              frame "F13" {
              }
              frame "F12" {
              }
              frame "F11" {
              }
              frame "F10" {
              }
              frame "F9" {
              }
              frame "F8" {
              }
              frame "F7" {
              }
              frame "F6" {
              }
              frame "F5" {
              }
              frame "F4" {
              }
              frame "F3" {
              }
              frame "F2" {
              }
              frame "F1" {
              }
              frame "Z" {
              }
              frame "Y" {
              }
              frame "X" {
              }
              frame "W" {
              }
              frame "V" {
              }
              frame "U" {
              }
              frame "T" {
              }
              frame "S" {
              }
              frame "R" {
              }
              frame "Q" {
              }
              frame "P" {
              }
              frame "O" {
              }
              frame "N" {
              }
              frame "M" {
              }
              frame "L" {
              }
              frame "K" {
              }
              frame "J" {
              }
              frame "I" {
              }
              frame "H" {
              }
              frame "G" {
              }
              frame "F" {
              }
              frame "E" {
              }
              frame "D" {
              }
              frame "C" {
              }
              frame "B" {
              }
              frame "A" {
              }
              frame "9" {
              }
              frame "8" {
              }
              frame "7" {
              }
              frame "6" {
              }
              frame "5" {
              }
              frame "4" {
              }
              frame "3" {
              }
              frame "2" {
              }
              frame "1" {
              }
              frame "0" {
              }
            }
            n90 = Bundle(w146, w147, w132, w133, 0.0) -> (w134:cluster{dbl, dbl, dbl, dbl, dbl})  [unwired: 1 in]
            n91 = Divide(x=20, y=w158) -> (x/y=w156:sgl)
            n92 = Bundle("X"=w126, "Y"=w127) -> (w130:cluster{"X":sgl, "Y":sgl})  [unwired: 1 in]
            n93 = call "IMAQ Convert Rectangle to ROI (Polygon)"("Rectangle"=w134) -> ("ROI Descriptor"=w136:T1)  [unwired: 7 in, 2 out]
            n94 = property on="Image Out" class="ImageControl"("Image Center Position"=w130) -> ()  [unwired: 2 in, 2 out]
            n95 = property on="Image Preview" class="ImageControl"("ROI"=w136) -> ()  [unwired: 2 in, 2 out]
            n96 = Bundle("Application Font", w156, w152, w152, w152, w152, w152, TRUE, w154) -> (w151:T18)  [unwired: 1 in]
            n97 = Bundle(w154, w151, w154, w154) -> (w106:T19)  [unwired: 1 in]
            n98 = local read "Image Out"() -> (w105:T9)
            n99 = property on="Image Out" class="ImageControl"() -> ("ZoomInteger"=w103:cluster{"X":i32, "Y":i32})  [unwired: 2 in, 2 out]
            n100 = property on="Image Out" class="ImageControl"() -> ("ROI"=w109:T13)  [unwired: 2 in, 2 out]
            n101 = Unbundle By Name(w109) -> ("Contours"=w110:T14)
            n102 = local read "No Image\n File"() -> (w99:path)
            n103 = local read "Image File"() -> (w98:path)
            n104 = call "IMAQ Clear Overlay"("Image"=w105) -> ("Image Out"=w124:T9)  [unwired: 9 in, 1 out]
            n105 = Initialize Array(0) -> (w112:i32[])  [unwired: 1 in]
            n106 = Array Size(array=w110) -> (size(s)=w111:i32)
            n107 = Unbundle(w103) -> ("X"=w102:i32)  [unwired: 1 out]
            n108 = Equal?(x=w99, y=w98) -> (x = y?=w97:bool)
            n109 = local write "Zoom"(w102) -> ()
            n110 = Build Array(0.505025, 0.252522, 0.127742, 0.050345, 0.031129) -> (w119:dbl[])
            n111 = local read "Magnification"() -> (w120:u16)
            n112 = Array Subset(array=w119, index=w120, length=1) -> (w122:dbl[])
            n113 = case shown="True" w97 {
              tunnel: w100 -> [w161 _]
              frame False {
                n114 = local write "Image Center X"(w161) -> ()
              }
              frame True {
              }
            }
            n115 = To Double Precision Float(number=w122) -> (double precision float=w123:dbl[])
            n116 = for {
              N: w111 -> [_]
              shift-right: [w206] -> _
              shift-left: w110 -> [w206]
              shift-right: [w182] -> w107
              shift-left: w112 -> [w204]
              tunnel: w123 -> [w203]
              shift-right: [w200] -> _
              shift-left: w124 -> [w202]
              tunnel: w106 -> [w196]
              i -> [w199]
              n117 = Index Array(array=w206, index=w199) -> (element=w215:T20)
              n118 = Unbundle(w215) -> ("Points"=w214:i32[])  [unwired: 2 out]
              n119 = Array To Cluster(array=w214) -> (cluster=w213:T21)
              n120 = Unbundle(w213) -> ("Points[0]"=w195:i32, "Points[1]"=w192:i32, "Points[2]"=w205:i32, "Points[3]"=w211:i32)  [unwired: 5 out]
              n121 = Add(x=w195, y=10) -> (x+y=w193:i32)
              n122 = Subtract(x=w192, y=w211) -> (x-y=w210:i32)
              n123 = Subtract(x=w195, y=w205) -> (x-y=w212:i32)
              n124 = Square(x=w210) -> (x^2=w208:i32)
              n125 = Square(x=w212) -> (x^2=w209:i32)
              n126 = Add(x=w209, y=w208) -> (x+y=w207:i32)
              n127 = Square Root(x=w207) -> (sqrt(x)=w186:dbl)
              n128 = Multiply(x=w186, y=0.5) -> (x*y=w189:dbl)
              n129 = Add(x=w189, y=w192) -> (x+y=w191:dbl)
              n130 = Bundle(w193, w191) -> (w201:cluster{i32, dbl})  [unwired: 1 in]
              n131 = Multiply(x=w186, y=w203) -> (x*y=w185:dbl[])
              n132 = Index Array(array=w185) -> (element=w198:dbl)  [unwired: 1 in]
              n133 = Number To Fractional String(number=w198, precision (6)=0) -> (F-format string=w197:string)  [unwired: 2 in]
              n134 = call "IMAQ Overlay Text"("BG Color (Transparent)"=u32 0, "Text Color (black)"=u32 16448250, "Font, Size & Style"=w196, "String"=w197, "Origin"=w201, "Image"=w202) -> ("Image Out"=w200:T9)  [unwired: 4 in, 1 out]
              n135 = Build Array (concatenate)(w204, w185) -> (w183:dbl[])
              n136 = To Long Integer(number=w183) -> (32bit integer=w182:i32[])
            }
            n137 = local write "Distances"(w107) -> ()
            n138 = Add Array Elements(numeric array=w107) -> (sum=w108:i32)
            n139 = local write "Total Width"(w108) -> ()
          }
        }
        n140 = Unbundle By Name(w89) -> ("Manual-Temp"=w94:bool, "Manual-Width"=w93:bool, "Manuel-Length"=w92:bool, "Manuel-Dielectric"=w91:bool, "Manual Comments"=w90:bool)
        n141 = stacked-sequence {
          tunnel: w94 -> [w556 _ _]
          tunnel: w93 -> [_ w565 _]
          tunnel: w92 -> [_ _ w581]
          tunnel: w91 -> [_ _ w578]
          tunnel: w90 -> [_ _ w577]
          frame #0 {
            n142 = local read "Rec: Temp"() -> (w555:dbl)
            n143 = case shown="True" w556 {
              tunnel: w555 -> [w561 _]
              frame False {
                n144 = local read "Rec: Temp"() -> (w559:dbl)
                n145 = property on="New: Temp" class="DigNum (strict)"("DisabledEnum"=1) -> ()  [unwired: 2 in, 2 out]
                n146 = Equal To 0?(x=w559) -> (x = 0?=w560:bool)
                n147 = local write "New: Temp"(w561) -> ()
                n148 = case shown="True" w560 {
                  tunnel: [w562 w563] -> w557
                  tunnel: w559 -> [w562 _]
                  frame False {
                  }
                  frame True {
                    n149 = local read "Room Temp"() -> (w563:dbl)
                  }
                }
                n150 = local write "Rec: Temp"(w557) -> ()
                n151 = local write "New: Temp"(w557) -> ()
              }
              frame True {
                n152 = property on="New: Temp" class="DigNum (strict)"("DisabledEnum"=0) -> ()  [unwired: 2 in, 2 out]
              }
            }
          }
          frame #1 {
            n153 = case shown="True" w565 {
              frame False {
                n154 = property on="New: Width" class="DigNum (strict)"("DisabledEnum"=1) -> ()  [unwired: 2 in, 2 out]
              }
              frame True {
                n155 = property on="New: Width" class="DigNum (strict)"("DisabledEnum"=0) -> ()  [unwired: 2 in, 2 out]
              }
            }
            n156 = local read "Total Width"() -> (w571:dbl)
            n157 = Equal To 0?(x=w571) -> (x = 0?=w568:bool)
            n158 = local read "Rec: Width"() -> (w569:dbl)
            n159 = Not(x=w565) -> (.not. x?=w567:bool)
            n160 = Or(x=w568, y=w565) -> (x .or. y?=w570:bool)
            n161 = And(x=w568, y=w567) -> (x .and. y?=w566:bool)
            n162 = case shown="True" w566 {
              tunnel: w569 -> [_ w574]
              frame False {
              }
              frame True {
                n163 = local write "New: Width"(w574) -> ()
              }
            }
            n164 = case shown="True" w570 {
              tunnel: w571 -> [w575 _]
              frame False {
                n165 = local write "New: Width"(w575) -> ()
              }
              frame True {
                n166 = property on="New: Width" class="DigNum (strict)"("DisabledEnum"=0) -> ()  [unwired: 2 in, 2 out]
              }
            }
          }
          frame #2 {
            n167 = local read "Rec: Length"() -> (w582:dbl)
            n168 = case shown="False" w581 {
              tunnel: w582 -> [w590 _]
              frame False {
                n169 = local write "New: Length"(w590) -> ()
                n170 = property on="New: Length" class="DigNum (strict)"("DisabledEnum"=1) -> ()  [unwired: 2 in, 2 out]
              }
              frame True {
                n171 = property on="New: Length" class="DigNum (strict)"("DisabledEnum"=0) -> ()  [unwired: 2 in, 2 out]
              }
            }
            n172 = local read "Comments:"() -> (w579:string)
            n173 = local read "Rec: Dielectric (d)"() -> (w580:dbl)
            n174 = case shown="False" w577 {
              tunnel: w579 -> [w584 _]
              frame False {
                n175 = local write "New: Comments"(w584) -> ()
                n176 = property on="New: Comments" class="Str"("DisabledEnum"=1) -> ()  [unwired: 2 in, 2 out]
              }
              frame True {
                n177 = property on="New: Comments" class="Str"("DisabledEnum"=0) -> ()  [unwired: 2 in, 2 out]
              }
            }
            n178 = case shown="False" w578 {
              tunnel: w580 -> [w587 _]
              frame False {
                n179 = local write "New: Dielectric"(w587) -> ()
                n180 = property on="New: Dielectric" class="DigNum (strict)"("DisabledEnum"=1) -> ()  [unwired: 2 in, 2 out]
              }
              frame True {
                n181 = property on="New: Dielectric" class="DigNum (strict)"("DisabledEnum"=0) -> ()  [unwired: 2 in, 2 out]
              }
            }
          }
        }
        n182 = property on="Next File" class="Bool (strict)"("Value"=w76) -> (error out=w85:errorcluster)  [unwired: 2 in, 1 out]
        n183 = property on="Previous File" class="Bool (strict)"(error in=w85, "Value"=w76) -> (error out=w84:errorcluster)  [unwired: 1 in, 1 out]
        n184 = property on="Save" class="Bool (strict)"(error in=w84, "Value"=w76) -> (error out=w83:errorcluster)  [unwired: 1 in, 1 out]
        n185 = property on="Export" class="Bool (strict)"("Value"=w76) -> ()  [unwired: 2 in, 2 out]
        n186 = property on="Save Next" class="Bool (strict)"(error in=w83, "Value"=w76) -> (error out=w82:errorcluster)  [unwired: 1 in, 1 out]
        n187 = property on="Discard" class="Bool (strict)"(error in=w82, "Value"=w76) -> (error out=w81:errorcluster)  [unwired: 1 in, 1 out]
        n188 = property on="Save Lines" class="Bool (strict)"(error in=w81, "Value"=w76) -> ()  [unwired: 1 in, 2 out]
        n189 = property on="Close" class="Bool (strict)"("Value"=w76) -> ()  [unwired: 2 in, 2 out]
        n190 = property on="Disable Flag" class="Bool (strict)"("Value"=w76) -> ()  [unwired: 2 in, 2 out]
        n191 = Cluster To Array(cluster=w75) -> (array=w95:bool[])
        n192 = call "Next State.vi"("Buttons []"=w95, "States []"=w96) -> ("Enum"=w88:T3)
        n193 = event shown="[12] \"Transfer File\": Value Change" {
          selector: _ -> [_ _ _ _ _ _ _ _ _ _ _ _ _]
          dyn-events: _ -> [_ _ _ _ _ _ _ _ _ _ _ _ _]
          timeout: 5 -> [_ _ _ _ _ _ _ _ _ _ _ _ _]
          tunnel: w88 -> [w435 _ _ _ _ _ _ _ _ _ _ _ _]
          tunnel: [w435 MegaAwesome_States."Re-Calculated Values" MegaAwesome_States."Re-Calculated Values" MegaAwesome_States."Re-Calculated Values" MegaAwesome_States."Re-Calculated Values" MegaAwesome_States."Calculated Values" MegaAwesome_States."Re-Calculated Values" MegaAwesome_States."Re-Calculated Values" MegaAwesome_States."Calculated Values" MegaAwesome_States."Re-Calculated Values" MegaAwesome_States."Re-Calculated Values" MegaAwesome_States."Read Data" MegaAwesome_States."Read Data"] -> w87
          tunnel: w79 -> [w434 w436 w438 w440 w442 w444 w446 w471 w496 w501 w525 _ w553]
          tunnel: [w434 w436 w438 w440 w442 w444 w446 w471 w496 w501 w525 w544 w553] -> w78
          tunnel: w77 -> [_ _ _ _ _ _ _ _ _ _ _ w543 _]
          tunnel: w75 -> [_ _ _ _ _ _ _ _ _ _ _ _ _]
          event Timeout {
            n194 = event-data() -> ()  [unwired: 1 in, 2 out]
          }
          event "New: Dielectric": Value Change {
            n195 = event-data() -> ()  [unwired: 1 in, 5 out]
          }
          event "New: Length": Value Change {
            n196 = event-data() -> ()  [unwired: 1 in, 5 out]
          }
          event "New: Width": Value Change {
            n197 = event-data() -> ()  [unwired: 1 in, 5 out]
          }
          event "New: Temp": Value Change {
            n198 = event-data() -> ()  [unwired: 1 in, 5 out]
          }
          event "Num Pts Log", "Transport Style Controls", "Num Pts": Value Change {
            n199 = event-data() -> ()  [unwired: 1 in, 5 out]
          }
          event "Sat-Trans Slider": Value Change {
            n200 = event-data() -> ()  [unwired: 1 in, 5 out]
            n201 = local read "Sqrt-Sat"() -> (w470:cluster{dbl[], dbl[]}[])
            n202 = Decimate 1D Array(w470) -> (w454:cluster{dbl[], dbl[]}[], w455:cluster{dbl[], dbl[]}[])
            n203 = local read "Slider Min"() -> (w451:dbl)
            n204 = local read "Sat-Trans Slider"() -> (w449:dbl)
            n205 = Array To Cluster(array=w454) -> (cluster=w469:T22)
            n206 = local read "New: Dielectric"() -> (w464:dbl)
            n207 = local read "Num Pts"() -> (w447:dbl)
            n208 = local read "New: Width"() -> (w466:dbl)
            n209 = local read "New: Length"() -> (w465:dbl)
            n210 = Unbundle(w469) -> ("[0]"=w468:cluster{dbl[], dbl[]})  [unwired: 8 out]
            n211 = Absolute Value(x=w451) -> (abs(x)=w450:dbl)
            n212 = Unbundle(w468) -> (w452:dbl[], w467:dbl[])
            n213 = Add(x=w449, y=w450) -> (x+y=w448:dbl)
            n214 = Array Subset(array=w452, index=w448, length=w447) -> (w462:dbl[])
            n215 = local write "Sat Vg Array-Used"(w462) -> ()
            n216 = Array Subset(array=w467, index=w448, length=w447) -> (w463:dbl[])
            n217 = call "Mobility-Vt-Used Pts_Saturation.vi"("Width"=w466, "Length"=w465, "Dielectric (d)"=w464, "Sat Id Used"=w463, "Vg Used"=w462) -> ("Vt"=w458:dbl, "Mobility"=w459:dbl)  [unwired: 4 in, 1 out]
            n218 = local write "Index-Sat"(w448) -> ()
            n219 = local write "Sat Id-Used"(w463) -> ()
            n220 = Bundle(w462, w463) -> (w456:cluster{dbl[], dbl[]})  [unwired: 1 in]
            n221 = local read "Re-Calculated Values Cluster"() -> (w461:T10)
            n222 = Bundle By Name(cluster=w461, "Mobility-Sat"=w459, "Vt-Sat"=w458) -> (w460:T10)
            n223 = local write "Re-Calculated Values Cluster"(w460) -> ()
            n224 = Build Array (concatenate)(w454, w455, w456) -> (w453:cluster{dbl[], dbl[]}[])
            n225 = local write "Sqrt-Sat"(w453) -> ()
          }
          event "Lin-Trans Slider": Value Change {
            n226 = event-data() -> ()  [unwired: 1 in, 5 out]
            n227 = local read "Sqrt-Lin"() -> (w495:cluster{dbl[], dbl[]}[])
            n228 = Decimate 1D Array(w495) -> (w480:cluster{dbl[], dbl[]}[], w481:cluster{dbl[], dbl[]}[])
            n229 = local read "Slider Min"() -> (w477:dbl)
            n230 = Array To Cluster(array=w480) -> (cluster=w494:T22)
            n231 = local read "Lin-Trans Slider"() -> (w475:dbl)
            n232 = local read "New: Dielectric"() -> (w488:dbl)
            n233 = local read "Num Pts"() -> (w491:dbl)
            n234 = local read "New: Width"() -> (w490:dbl)
            n235 = local read "New: Length"() -> (w489:dbl)
            n236 = local read "Lin Vd"() -> (w472:dbl)
            n237 = Unbundle(w494) -> ("[0]"=w493:cluster{dbl[], dbl[]})  [unwired: 8 out]
            n238 = Absolute Value(x=w477) -> (abs(x)=w476:dbl)
            n239 = Unbundle(w493) -> (w478:dbl[], w492:dbl[])
            n240 = Add(x=w475, y=w476) -> (x+y=w474:dbl)
            n241 = Array Subset(array=w478, index=w474, length=w491) -> (w486:dbl[])
            n242 = local write "Lin-Vg Array-Used"(w486) -> ()
            n243 = Array Subset(array=w492, index=w474, length=w491) -> (w487:dbl[])
            n244 = call "Mobility-Vt-Used Pts_Linear.vi"("Width"=w490, "Length"=w489, "Vd"=w472, "Dielectric (d)"=w488, "Id Used"=w487, "Vg Used"=w486) -> ("Mobility"=w483:dbl)  [unwired: 3 in, 2 out]
            n245 = local write "Index-Lin"(w474) -> ()
            n246 = local write "Lin Id-Used"(w487) -> ()
            n247 = Bundle(w486, w487) -> (w482:cluster{dbl[], dbl[]})  [unwired: 1 in]
            n248 = local read "Re-Calculated Values Cluster"() -> (w485:T10)
            n249 = Bundle By Name(cluster=w485, "Moblitity-Lin"=w483) -> (w484:T10)
            n250 = local write "Re-Calculated Values Cluster"(w484) -> ()
            n251 = Build Array (concatenate)(w480, w481, w482) -> (w479:cluster{dbl[], dbl[]}[])
            n252 = local write "Sqrt-Lin"(w479) -> ()
          }
          event "Image Analysis", "1) Transport": Value Change {
            n253 = event-data() -> ()  [unwired: 1 in, 5 out]
          }
          event "Sat-Log Slider": Value Change {
            n254 = event-data() -> ()  [unwired: 1 in, 5 out]
            n255 = local read "Sat-Log"() -> (w504:cluster{dbl[], dbl[]}[])
            n256 = property on="Sat-Log" class="XYGraph (strict)"("Active Plot"=2, "Plot.Fill/Pt. Color"=u32 6618880, "Plot.Point Style"=11) -> ()  [unwired: 2 in, 2 out]
            n257 = Decimate 1D Array(w504) -> (w511:cluster{dbl[], dbl[]}[], w512:cluster{dbl[], dbl[]}[])
            n258 = local read "Slider Min"() -> (w508:dbl)
            n259 = Array To Cluster(array=w511) -> (cluster=w521:T22)
            n260 = local read "Num Pts Log"() -> (w518:dbl)
            n261 = local read "Sat-Log Slider"() -> (w506:dbl)
            n262 = Unbundle(w521) -> ("[0]"=w520:cluster{dbl[], dbl[]})  [unwired: 8 out]
            n263 = Absolute Value(x=w508) -> (abs(x)=w507:dbl)
            n264 = Unbundle(w520) -> (w509:dbl[], w519:dbl[])
            n265 = Add(x=w506, y=w507) -> (x+y=w503:dbl)
            n266 = Array Subset(array=w509, index=w503, length=w518) -> (w516:dbl[])
            n267 = Array Subset(array=w519, index=w503, length=w518) -> (w517:dbl[])
            n268 = local write "Vg Array-Log-Used"(w516) -> ()
            n269 = local write "IndexLog-Sat"(w503) -> ()
            n270 = Bundle(w516, w517) -> (w502:cluster{dbl[], dbl[]})  [unwired: 1 in]
            n271 = call "STS-Used.vi"("Id Used"=w517, "Vg-Used"=w516) -> ("STS"=w513:dbl)  [unwired: 9 in]
            n272 = local write "Sat Id-Log-Used"(w517) -> ()
            n273 = local read "Re-Calculated Values Cluster"() -> (w515:T10)
            n274 = Bundle By Name(cluster=w515, "STS"=w513) -> (w514:T10)
            n275 = local write "Re-Calculated Values Cluster"(w514) -> ()
            n276 = Build Array (concatenate)(w511, w512, w502) -> (w510:cluster{dbl[], dbl[]}[])
            n277 = local write "Sat-Log"(w510) -> ()
          }
          event "Lin-Log Slider": Value Change {
            # "No Indicator for Lin-Log Slider Use"
            n278 = event-data() -> ()  [unwired: 1 in, 5 out]
            n279 = local read "Lin-Log"() -> (w529:cluster{dbl[], dbl[]}[])
            n280 = property on="Lin-Log" class="XYGraph (strict)"("Active Plot"=2, "Plot.Fill/Pt. Color"=u32 6618880, "Plot.Point Style"=11) -> ()  [unwired: 2 in, 2 out]
            n281 = Decimate 1D Array(w529) -> (w535:cluster{dbl[], dbl[]}[], w536:cluster{dbl[], dbl[]}[])
            n282 = local read "Slider Min"() -> (w532:dbl)
            n283 = Array To Cluster(array=w535) -> (cluster=w542:T22)
            n284 = local read "Num Pts Log"() -> (w539:dbl)
            n285 = local read "Lin-Log Slider"() -> (w530:dbl)
            n286 = Unbundle(w542) -> ("[0]"=w541:cluster{dbl[], dbl[]})  [unwired: 8 out]
            n287 = Absolute Value(x=w532) -> (abs(x)=w531:dbl)
            n288 = Unbundle(w541) -> (w533:dbl[], w540:dbl[])
            n289 = Add(x=w530, y=w531) -> (x+y=w528:dbl)
            n290 = Array Subset(array=w533, index=w528, length=w539) -> (w537:dbl[])
            n291 = local write "Lin-Vg Array-Log Used"(w537) -> ()
            n292 = Array Subset(array=w540, index=w528, length=w539) -> (w538:dbl[])
            n293 = local write "IndexLog-Sat"(w528) -> ()
            n294 = Bundle(w537, w538) -> (w527:cluster{dbl[], dbl[]})  [unwired: 1 in]
            n295 = local write "Lin Id-Log Used"(w538) -> ()
            n296 = Build Array (concatenate)(w535, w536, w527) -> (w534:cluster{dbl[], dbl[]}[])
            n297 = local write "Lin-Log"(w534) -> ()
          }
          event "Index Array": Value Change {
            n298 = event-data() -> ()  [unwired: 1 in, 5 out]
            n299 = Strip Path(path=w543) -> (stripped path=w549:path)  [unwired: 1 out]
            n300 = local write "Transfer Folder"(w549) -> ()
            n301 = List Folder(path=w549) -> (filenames=w545:string[])  [unwired: 3 in, 3 out]
            n302 = local read "Index Array"() -> (w544:u16)
            n303 = Path To String(path=w549) -> (string=w550:string)
            n304 = Index Array(array=w545, index=w544) -> (element=w551:string)
            n305 = Concatenate Strings(w550, "\\", w551) -> (w547:string)
            n306 = String To Path(string=w547) -> (path=w546:path)
            n307 = local write "Transfer File"(w546) -> ()
          }
          event "Transfer File": Value Change {
            n308 = event-data() -> ()  [unwired: 1 in, 5 out]
          }
        }
      }
      frame "Read Data" {
        n309 = call "IMAQ Dispose"("All Images? (No)"=TRUE) -> ()  [unwired: 5 in, 1 out]
        n310 = case shown="False" "Disable Flag" {
          tunnel: w598 -> [_ w625]
          tunnel: [w621 w622] -> w597
          tunnel: w595 -> [w621 _]
          frame False {
          }
          frame True {
            n311 = local read "Transfer Folder"() -> (w624:path)
            n312 = List Folder(path=w624) -> (filenames=w626:string[])  [unwired: 3 in, 3 out]
            n313 = Index Array(array=w626, index=w625) -> (element=w623:string)
            n314 = Build Path(base path=w624, name or relative path=w623) -> (appended path=w622:path)
            n315 = local write "Transfer File"(w622) -> ()
          }
        }
        n316 = call "Recorded Values.vi"("Path"=w597) -> ("Recorded Char"=w620:T10, "Recorded Prop"=w611:T2, "Fabrication Prop"=w609:T5)  [unwired: 8 in]
        n317 = Strip Path(path=w597) -> (stripped path=w608:path, name=w607:string)
        n318 = local write "Fabrication Prop"(w609) -> ()
        n319 = local write "Recorded Prop"(w611) -> ()
        n320 = Unbundle By Name(w611) -> ("Date Recorded"=w593:string, "Index"=w610:string, "Length"=w603:dbl, "Width"=w602:dbl)  [unwired: 1 out]
        n321 = local write "Recorded Values Cluster"(w620) -> ()
        n322 = Unbundle By Name(w611) -> ("Sample Temp"=w613:dbl)
        n323 = Unbundle By Name(w609) -> ("Dielectric (nm)"=w604:dbl, "Comments"=w605:string, "Date Created"=w594:string)
        n324 = List Folder(path=w608) -> (filenames=w601:string[])  [unwired: 3 in, 3 out]
        n325 = local write "Rec: Dielectric (d)"(w604) -> ()
        n326 = local write "Date Created"(w594) -> ()
        n327 = local write "Index"(w610) -> ()
        n328 = local write "Rec: Length"(w603) -> ()
        n329 = local write "Rec: Width"(w602) -> ()
        n330 = Equal To 0?(x=w613) -> (x = 0?=w616:bool)
        n331 = Number To Decimal String(number=w613) -> (decimal integer string=w617:string)  [unwired: 1 in]
        n332 = local write "Comments:"(w605) -> ()
        n333 = Search 1D Array(1D array=w601, element=w607) -> (index of element=w600:i32)  [unwired: 1 in]
        n334 = Equal?(x="", y=w617) -> (x = y?=w615:bool)
        n335 = Index Array(array=w601, index=w600) -> (element=w606:string)
        n336 = local write "New: Width"(w602) -> ()
        n337 = local write "New: Length"(w603) -> ()
        n338 = local write "Index Array"(w600) -> ()
        n339 = local write "Date Recorded"(w593) -> ()
        n340 = Or(x=w616, y=w615) -> (x .or. y?=w614:bool)
        n341 = local write "New: Dielectric"(w604) -> ()
        n342 = local write "Data Name:"(w606) -> ()
        n343 = case shown="True" w614 {
          tunnel: [w627 w628] -> w592
          tunnel: w613 -> [w627 _]
          frame False {
          }
          frame True {
            n344 = local read "Room Temp"() -> (w628:dbl)
          }
        }
        n345 = local write "New: Temp"(w592) -> ()
        n346 = Bundle By Name(cluster=w611, "Sample Temp"=w592) -> (w612:T2)
        n347 = local write "Rec: Temp"(w592) -> ()
        n348 = local write "Recorded Prop"(w612) -> ()
      }
      frame "Calculated Values" {
        n349 = case shown="True" w633 {
          selector: w633 -> [w706 _]
          tunnel: w642 -> [w705 w717]
          tunnel: w631 -> [w704 w713]
          tunnel: w630 -> [w709 w711]
          frame False {
            n350 = call "TRF to TSP Plot_09_21_12a_JW.vi"("Plot Transport"=w706, "No Transport File"=w709, "Transport Folder"=w704, "Transfer File"=w705) -> ("Transport"=w707:cluster{ext[], ext[]}[], "Transport File"=w708:path, "Transport Name"=w703:string)  [unwired: 5 in]
            n351 = local write "Transport"(w707) -> ()
            n352 = local write "Transport\nFile"(w708) -> ()
            n353 = local write "Transport Name:"(w703) -> ()
          }
          frame True {
            n354 = local read "Transport Style Controls"() -> (w716:T11)
            n355 = call "TRF to TSP Plot_09_21_12a_JW.vi"("Transport Graph Properties"=w716, "No Transport File"=w711, "Transport Folder"=w713, "Transfer File"=w717) -> ("Transport"=w715:cluster{ext[], ext[]}[], "Transport File"=w712:path, "Transport Name"=w710:string)  [unwired: 5 in]
            n356 = Array Size(array=w715) -> (size(s)=w714:i32)
            n357 = local write "Transport"(w715) -> ()
            n358 = for {
              N: w714 -> [_]
              tunnel: w716 -> [w721]
              i -> [w720]
              n359 = Unbundle By Name(w721) -> ("Transport Line Size"=w718:u16, "Transport Line Color"=w719:u32)
              n360 = property on="Transport" class="XYGraph (strict)"("Active Plot"=w720, "Plot.Plot Color"=w719, "Plot.Line Width"=w718) -> ()  [unwired: 2 in, 2 out]
            }
            n361 = local write "Transport\nFile"(w712) -> ()
            n362 = local write "Transport Name:"(w710) -> ()
          }
        }
        n363 = case shown="True" w632 {
          tunnel: w662 -> [_ w691]
          tunnel: w661 -> [w683 w697]
          tunnel: w642 -> [_ w696]
          frame False {
            n364 = call "Vision Acquisition2"("Image Path"=w683) -> ("Image Out"=w682:T9)  [unwired: 25 in, 1 out]
            n365 = local write "Image Out"(w682) -> ()
            n366 = local write "Image Preview"(w682) -> ()
          }
          frame True {
            n367 = local read "Image Center X"() -> (w684:i32)
            n368 = call "Image from TRF Display.vi"("Image Center X"=w684, "No Image File"=w697, "Image Folder"=w691, "Transfer File"=w696) -> ("Image Preview"=w692:T9, "Image Out"=w693:T9, "Image File"=w694:path, "Image Name"=w695:string, "ROI File"=w688:path)  [unwired: 3 in]
            n369 = invoke on="Image Out" class="ImageControl" method="Clear ROI"() -> ()  [unwired: 3 in, 3 out]
            n370 = local write "Image File"(w694) -> ()
            n371 = local write "Image Name"(w695) -> ()
            n372 = local write "Image Out"(w693) -> ()
            n373 = local write "Image Preview"(w692) -> ()
            n374 = call <vilib>:"Check if File or Folder Exists.vi"("path"=w688) -> ("file or folder exists?"=w689:bool, "dup path"=w690:path)  [unwired: 8 in, 1 out]
            n375 = case shown="True" w689 {
              tunnel: w690 -> [_ w698]
              frame False {
              }
              frame True {
                n376 = Read from Text File(file (use dialog)=w698) -> (text=w702:string)  [unwired: 3 in, 3 out]
                n377 = property on="Image Out" class="ImageControl"() -> ("ROI"=w699:T13)  [unwired: 2 in, 2 out]
                n378 = Unflatten From String(type=w699, binary string=w702) -> (value=w700:T13, error out=w701:errorcluster)  [unwired: 3 in, 1 out]
                n379 = property on="Image Out" class="ImageControl"(error in=w701, "ROI"=w700) -> ()  [unwired: 1 in, 2 out]
              }
            }
            n380 = local read "Image Center X"() -> (w685:i32)
            n381 = Bundle("Image Center X"=w685, 0) -> (w687:cluster{"Image Center X":i32, i32})  [unwired: 1 in]
            n382 = property on="Image Out" class="ImageControl"("Image Center Position"=w687) -> ()  [unwired: 2 in, 2 out]
          }
        }
        n383 = local read "Recorded Prop"() -> (w664:T2)
        n384 = local read "Fabrication Prop"() -> (w671:T5)
        n385 = local read "Calculated Values Cluster"() -> (w681:T10)
        n386 = call "Mobility-Vt Calculator-File.vi"("NumPts"=w666, "Path"=w642) -> ("Used Points"=w659:T23, "Graph Cluster"=w648:T24, "Lin Vd"=w655:dbl, "Output"=w679:T25)  [unwired: 6 in]
        n387 = call "STS Calculator-File.vi"("NumPts"=w665, "Path"=w642) -> ("Used Points"=w653:T26, "XY Graph-Sat"=w636:cluster{dbl[], dbl[]}[], "XY Graph-Lin"=w629:cluster{dbl[], dbl[]}[], "Ouput"=w674:cluster{"STS-Sat":dbl, "STS-Lin":dbl})  [unwired: 6 in]
        n388 = Unbundle By Name(w671) -> ("Dielectric (nm)"=w669:dbl)
        n389 = Unbundle By Name(w664) -> ("Sample Temp"=w663:dbl)
        n390 = Unbundle By Name(w679) -> ("Mobility-Sat"=w678:dbl, "Vt-Sat"=w670:dbl, "Mobility-Lin"=w677:dbl, "Off I-Sat"=w676:dbl, "On/Off I-Sat"=w675:dbl)  [unwired: 1 out]
        n391 = local write "Lin Vd"(w655) -> ()
        n392 = Unbundle By Name(w674) -> ("STS-Sat"=w668:dbl)  [unwired: 1 out]
        n393 = local write "Sat-Log"(w636) -> ()
        n394 = local write "Lin-Log"(w629) -> ()
        n395 = call "Trap Density_VT.vi"("VT"=w670, "Dielectric"=w669) -> ("Trap Density-VT"=w673:dbl)
        n396 = call "Trap Density_STS.vi"("Temp (T) [K]"=w663, "S.T.S. (S)"=w668, "Dielectric"=w669) -> ("Trap Density (N)"=w672:dbl)  [unwired: 8 in]
        n397 = Bundle By Name(cluster=w681, "Mobility-Sat"=w678, "Moblitity-Lin"=w677, "On/Off"=w675, "Off Current"=w676, "Vt-Sat"=w670, "STS"=w668, "Trap Density-VT"=w673, "Trap Density-STS"=w672) -> (w680:T10)
        n398 = Unbundle By Name(w653) -> ("Sat Vg Used"=w652:dbl[], "Sat Log(Id) Used"=w651:dbl[], "Lin Vg Used"=w650:dbl[], "Lin Log(Id) Used"=w649:dbl[], "STS Index-Sat"=w634:dbl, "STS Index-Lin"=w635:dbl)
        n399 = Unbundle By Name(w659) -> ("Sat Vg Used"=w658:dbl[], "Sat Sqrt(Id) Used"=w657:dbl[], "Lin Vg Used"=w656:dbl[], "Lin Sqrt(Id) Used"=w654:dbl[], "Index-Lin"=w644:dbl, "Index-Sat"=w643:dbl)
        n400 = local write "Vg Array-Log-Used"(w652) -> ()
        n401 = local write "Sat Id-Log-Used"(w651) -> ()
        n402 = local write "Lin-Vg Array-Log Used"(w650) -> ()
        n403 = local write "Lin Id-Log Used"(w649) -> ()
        n404 = local write "IndexLog-Sat"(w634) -> ()
        n405 = local write "Index-Lin"(w635) -> ()
        n406 = local write "Calculated Values Cluster"(w680) -> ()
        n407 = local write "Sat Vg Array-Used"(w658) -> ()
        n408 = local write "Sat Id-Used"(w657) -> ()
        n409 = local write "Lin-Vg Array-Used"(w656) -> ()
        n410 = local write "Lin Id-Used"(w654) -> ()
        n411 = local write "Index-Sat"(w643) -> ()
        n412 = local write "Index-Lin"(w644) -> ()
        n413 = local write "Lin-Log Slider"(w635) -> ()
        n414 = local write "Sat-Log Slider"(w634) -> ()
        n415 = local write "Sat-Trans Slider"(w643) -> ()
        n416 = local write "Lin-Trans Slider"(w644) -> ()
        n417 = Unbundle By Name(w648) -> ("Raw Sat"=w641:cluster{dbl[], dbl[]}[], "Sqrt Sat"=w645:cluster{dbl[], dbl[]}[], "Raw Lin"=w647:cluster{dbl[], dbl[]}[], "Sqrt Lin"=w646:cluster{dbl[], dbl[]}[])
        n418 = Index Array(array=w641) -> (element=w640:cluster{dbl[], dbl[]})  [unwired: 1 in]
        n419 = Unbundle(w640) -> (w639:dbl[])  [unwired: 1 out]
        n420 = Array Max & Min(array=w639) -> (max value=w638:dbl, min value=w637:dbl)  [unwired: 2 out]
        n421 = property on="Sat-Trans Slider" class="Slide (strict)"("Scale.Maximum"=w638, "Scale.Minimum"=w637) -> ()  [unwired: 2 in, 2 out]
        n422 = property on="Lin-Trans Slider" class="Slide (strict)"("Scale.Maximum"=w638, "Scale.Minimum"=w637) -> ()  [unwired: 2 in, 2 out]
        n423 = property on="Sat-Log Slider" class="Slide (strict)"("Scale.Maximum"=w638, "Scale.Minimum"=w637) -> ()  [unwired: 2 in, 2 out]
        n424 = property on="Lin-Log Slider" class="Slide (strict)"("Scale.Maximum"=w638, "Scale.Minimum"=w637) -> ()  [unwired: 2 in, 2 out]
        n425 = local write "Slider Max"(w638) -> ()
        n426 = local write "Slider Min"(w637) -> ()
        n427 = local write "Raw- Sat"(w641) -> ()
        n428 = local write "Raw- Lin"(w647) -> ()
        n429 = local write "Sqrt-Sat"(w645) -> ()
        n430 = local write "Sqrt-Lin"(w646) -> ()
      }
      frame "Re-Calculated Values" {
        n431 = local read "Vg Array-Log-Used"() -> (w730:dbl[])
        n432 = local read "Sat Vg Array-Used"() -> (w738:dbl[])
        n433 = local read "Lin-Vg Array-Used"() -> (w744:dbl[])
        n434 = local read "Sat Id-Log-Used"() -> (w729:dbl[])
        n435 = local read "New: Dielectric"() -> (w742:dbl)
        n436 = local read "New: Dielectric"() -> (w727:dbl)
        n437 = local read "New: Length"() -> (w741:dbl)
        n438 = local read "New: Length"() -> (w737:dbl)
        n439 = local read "New: Width"() -> (w740:dbl)
        n440 = local read "New: Width"() -> (w736:dbl)
        n441 = local read "Lin Id-Used"() -> (w743:dbl[])
        n442 = local read "Sat Id-Used"() -> (w735:dbl[])
        n443 = local read "Re-Calculated Values Cluster"() -> (w746:T10)
        n444 = local read "New: Dielectric"() -> (w726:dbl)
        n445 = local read "New: Temp"() -> (w725:dbl)
        n446 = local read "Lin Vd"() -> (w722:dbl)
        n447 = call "Mobility-Vt-Used Pts_Saturation.vi"("Width"=w736, "Length"=w737, "Dielectric (d)"=w727, "Sat Id Used"=w735, "Vg Used"=w738) -> ("Vt"=w733:dbl, "Mobility"=w734:dbl)  [unwired: 4 in, 1 out]
        n448 = call "STS-Used.vi"("Id Used"=w729, "Vg-Used"=w730) -> ("STS"=w728:dbl)  [unwired: 9 in]
        n449 = call "Mobility-Vt-Used Pts_Linear.vi"("Width"=w740, "Length"=w741, "Vd"=w722, "Dielectric (d)"=w742, "Id Used"=w743, "Vg Used"=w744) -> ("Mobility"=w739:dbl)  [unwired: 3 in, 2 out]
        n450 = call "Trap Density_VT.vi"("VT"=w733, "Dielectric"=w727) -> ("Trap Density-VT"=w732:dbl)
        n451 = call "Trap Density_STS.vi"("Temp (T) [K]"=w725, "S.T.S. (S)"=w728, "Dielectric"=w726) -> ("Trap Density (N)"=w724:dbl)  [unwired: 8 in]
        n452 = Bundle By Name(cluster=w746, "Mobility-Sat"=w734, "Moblitity-Lin"=w739, "Vt-Sat"=w733, "STS"=w728, "Trap Density-VT"=w732, "Trap Density-STS"=w724) -> (w745:T10)
        n453 = local write "Re-Calculated Values Cluster"(w745) -> ()
      }
      frame "Next File" {
        n454 = call "IMAQ Dispose"("All Images? (No)"=TRUE) -> ()  [unwired: 5 in, 1 out]
        n455 = Strip Path(path=w763) -> (stripped path=w754:path, name=w761:string)
        n456 = local write "Transfer Folder"(w754) -> ()
        n457 = List Folder(path=w754) -> (filenames=w748:string[])  [unwired: 3 in, 3 out]
        n458 = Array Size(array=w748) -> (size(s)=w760:i32)
        n459 = Search 1D Array(1D array=w748, element=w761) -> (index of element=w758:i32)  [unwired: 1 in]
        n460 = Decrement(x=w760) -> (x-1=w759:i32)
        n461 = Equal?(x=w759, y=w758) -> (x = y?=w757:bool)
        n462 = case shown="True" w757 {
          tunnel: w750 -> [w765 _]
          tunnel: [w764 0] -> w749
          frame False {
            n463 = Increment(x=w765) -> (x+1=w764:i32)
          }
          frame True {
          }
        }
        n464 = Path To String(path=w754) -> (string=w755:string)
        n465 = Index Array(array=w748, index=w749) -> (element=w756:string)
        n466 = Concatenate Strings(w755, "\\", w756) -> (w752:string)
        n467 = String To Path(string=w752) -> (path=w751:path)
        n468 = local write "Transfer File"(w751) -> ()
      }
      frame "Previous File" {
        n469 = call "IMAQ Dispose"("All Images? (No)"=TRUE) -> ()  [unwired: 5 in, 1 out]
        n470 = Strip Path(path=w774) -> (stripped path=w771:path, name=w782:string)
        n471 = local write "Transfer Folder"(w771) -> ()
        n472 = List Folder(path=w771) -> (filenames=w775:string[])  [unwired: 3 in, 3 out]
        n473 = Array Size(array=w775) -> (size(s)=w769:i32)
        n474 = Search 1D Array(1D array=w775, element=w782) -> (index of element=w781:i32)  [unwired: 1 in]
        n475 = Decrement(x=w769) -> (x-1=w768:i32)
        n476 = Equal To 0?(x=w781) -> (x = 0?=w780:bool)
        n477 = case shown="True" w780 {
          tunnel: w773 -> [w785 _]
          tunnel: [w784 w786] -> w772
          tunnel: w768 -> [_ w786]
          frame False {
            n478 = Decrement(x=w785) -> (x-1=w784:i32)
          }
          frame True {
          }
        }
        n479 = Path To String(path=w771) -> (string=w770:string)
        n480 = Index Array(array=w775, index=w772) -> (element=w779:string)
        n481 = Concatenate Strings(w770, "\\", w779) -> (w777:string)
        n482 = String To Path(string=w777) -> (path=w776:path)
        n483 = local write "Transfer File"(w776) -> ()
      }
      frame "Discard File" {
        n484 = flat-sequence {
          tunnel: w792 -> [w795]
          tunnel: [w795] -> w791
          tunnel: [w794] -> w788
          tunnel: w791 -> [w807]
          tunnel: w788 -> [w800]
          tunnel: [w799] -> w787
          frame #0 {
            n485 = Strip Path(path=w795) -> (stripped path=w798:path, name=w797:string)
            n486 = List Folder(path=w798) -> (filenames=w796:string[])  [unwired: 3 in, 3 out]
            n487 = Search 1D Array(1D array=w796, element=w797) -> (index of element=w794:i32)  [unwired: 1 in]
          }
          frame #1 {
            n488 = Strip Path(path=w807) -> (stripped path=w808:path, name=w806:string)
            n489 = String Subset(string=w806, offset (0)=0, length (rest)=1) -> (substring=w803:string)
            n490 = Equal?(x=w803, y="X") -> (x = y?=w801:bool)
            n491 = case shown="True" w801 {
              tunnel: w808 -> [w815 _]
              tunnel: w807 -> [w811 _]
              tunnel: w806 -> [w810 _]
              tunnel: w800 -> [w809 w819]
              tunnel: [w809 w818] -> w799
              frame False {
                n492 = Path To String(path=w815) -> (string=w814:string)
                n493 = Concatenate Strings(w814, "\\", "X_", w810) -> (w813:string)
                n494 = String To Path(string=w813) -> (path=w812:path)
                n495 = Move(source path=w811, 10:w812) -> ()  [unwired: 3 in, 3 out]
              }
              frame True {
                n496 = Increment(x=w819) -> (x+1=w818:i32)
              }
            }
          }
        }
        n497 = property on="Disable Flag" class="Bool (strict)"("Value"=TRUE) -> ()  [unwired: 2 in, 2 out]
        n498 = call "IMAQ Dispose"("All Images? (No)"=TRUE) -> ()  [unwired: 5 in, 1 out]
      }
      frame "Save" {
        n499 = stacked-sequence {
          seq-local: [w835 _] -> [_ w1332]
          seq-local: [w834 _] -> [_ w1330]
          tunnel: w827 -> [w836 w1333]
          frame #0 {
            # "Saves each Re-calculated parameter in sequence"
            n500 = stacked-sequence {
              tunnel: [_ _ _ _ _ _ _ _ _ _ _ _ _ w1300] -> w834
              tunnel: w836 -> [w856 _ _ _ _ _ _ _ _ _ _ _ _ _]
              frame #0 {
                n501 = call-poly <vilib>:"Read From Spreadsheet File.vi"("file path (dialog if empty)"=w856) -> ("all rows"=w855:string[][])  [unwired: 6 in, 4 out]
                n502 = Array Size(array=w855) -> (size(s)=w860:i32[])
                n503 = Array Subset(array=w855, index (row)=0, index (col)=0, length (col)=3) -> (w864:string[][])  [unwired: 1 in]
                n504 = Index Array(array=w860, index=0) -> (element=w858:i32)
                n505 = Reshape Array(w864, w858) -> (w857:string[])
                n506 = Search 1D Array(1D array=w857, element="Dielectric (nm):") -> (index of element=w867:i32)  [unwired: 1 in]
                n507 = Equal?(x=w867, y=-1) -> (x = y?=w866:bool)
                n508 = case shown="False" w866 {
                  tunnel: w855 -> [w875 w879]
                  tunnel: w867 -> [w871 _]
                  tunnel: [w870 w879] -> w865
                  frame False {
                    n509 = local read "Rec: Dielectric (d)"() -> (w877:dbl)
                    n510 = Number To Fractional String(number=w877) -> (F-format string=w872:string)  [unwired: 3 in]
                    n511 = Divide(x=w871, y=3) -> (x/y=w874:dbl)
                    n512 = To Word Integer(number=w874) -> (16bit integer=w873:i16)
                    n513 = Replace Array Subset(array=w875, new element=w872, index (row)=w873, index (col)=1) -> (w870:string[][])
                  }
                  frame True {
                  }
                }
                n514 = local write "Save Array"(w865) -> ()
              }
              frame #1 {
                n515 = local read "Save Array"() -> (w881:string[][])
                n516 = Array Size(array=w881) -> (size(s)=w884:i32[])
                n517 = Array Subset(array=w881, index (row)=0, index (col)=0, length (col)=3) -> (w888:string[][])  [unwired: 1 in]
                n518 = Index Array(array=w884, index=0) -> (element=w882:i32)
                n519 = Reshape Array(w888, w882) -> (w880:string[])
                n520 = Search 1D Array(1D array=w880, element="Comments:") -> (index of element=w891:i32)  [unwired: 1 in]
                n521 = Equal?(x=w891, y=-1) -> (x = y?=w890:bool)
                n522 = case shown="False" w890 {
                  tunnel: w881 -> [w899 w902]
                  tunnel: w891 -> [w896 _]
                  tunnel: [w895 w902] -> w889
                  frame False {
                    n523 = local read "New: Comments"() -> (w894:string)
                    n524 = Divide(x=w896, y=3) -> (x/y=w898:dbl)
                    n525 = To Word Integer(number=w898) -> (16bit integer=w897:i16)
                    n526 = Replace Array Subset(array=w899, new element=w894, index (row)=w897, index (col)=1) -> (w895:string[][])
                  }
                  frame True {
                  }
                }
                n527 = local write "Save Array"(w889) -> ()
              }
              frame #2 {
                n528 = local read "Save Array"() -> (w904:string[][])
                n529 = Array Size(array=w904) -> (size(s)=w907:i32[])
                n530 = Array Subset(array=w904, index (row)=0, index (col)=0, length (col)=3) -> (w911:string[][])  [unwired: 1 in]
                n531 = Index Array(array=w907, index=0) -> (element=w905:i32)
                n532 = Reshape Array(w911, w905) -> (w903:string[])
                n533 = Search 1D Array(1D array=w903, element="Length (um):") -> (index of element=w914:i32)  [unwired: 1 in]
                n534 = Equal?(x=w914, y=-1) -> (x = y?=w913:bool)
                n535 = case shown="False" w913 {
                  tunnel: w904 -> [w924 w927]
                  tunnel: w914 -> [w921 _]
                  tunnel: [w920 w927] -> w912
                  frame False {
                    n536 = local read "New: Length"() -> (w917:dbl)
                    n537 = Divide(x=w921, y=3) -> (x/y=w923:dbl)
                    n538 = Format Value(format string="%#g", value (0)=w917) -> (output string=w918:string)  [unwired: 1 in]
                    n539 = To Word Integer(number=w923) -> (16bit integer=w922:i16)
                    n540 = Replace Array Subset(array=w924, new element=w918, index (row)=w922, index (col)=1) -> (w920:string[][])
                  }
                  frame True {
                  }
                }
                n541 = local write "Save Array"(w912) -> ()
              }
              frame #3 {
                n542 = local read "Save Array"() -> (w929:string[][])
                n543 = Array Size(array=w929) -> (size(s)=w934:i32[])
                n544 = Array Subset(array=w929, index (row)=0, index (col)=0, length (col)=3) -> (w930:string[][])  [unwired: 1 in]
                n545 = Index Array(array=w934, index=0) -> (element=w936:i32)
                n546 = Reshape Array(w930, w936) -> (w928:string[])
                n547 = Search 1D Array(1D array=w928, element="Width (um):") -> (index of element=w939:i32)  [unwired: 1 in]
                n548 = Equal?(x=w939, y=-1) -> (x = y?=w938:bool)
                n549 = case shown="False" w938 {
                  tunnel: w939 -> [w947 _]
                  tunnel: w929 -> [w946 w952]
                  tunnel: [w945 w952] -> w937
                  frame False {
                    n550 = local read "New: Width"() -> (w942:dbl)
                    n551 = Divide(x=w947, y=3) -> (x/y=w949:dbl)
                    n552 = To Word Integer(number=w949) -> (16bit integer=w948:i16)
                    n553 = Format Value(format string="%#g", value (0)=w942) -> (output string=w943:string)  [unwired: 1 in]
                    n554 = Replace Array Subset(array=w946, new element=w943, index (row)=w948, index (col)=1) -> (w945:string[][])
                  }
                  frame True {
                  }
                }
                n555 = local write "Save Array"(w937) -> ()
              }
              frame #4 {
                w962 = "Sample Temp (K):"
                n556 = local read "Save Array"() -> (w954:string[][])
                n557 = Array Size(array=w954) -> (size(s)=w959:i32[])
                n558 = Array Subset(array=w954, index (row)=0, index (col)=0, length (col)=3) -> (w955:string[][])  [unwired: 1 in]
                n559 = Index Array(array=w959, index=0) -> (element=w961:i32)
                n560 = Reshape Array(w955, w961) -> (w953:string[])
                n561 = Search 1D Array(1D array=w953, element=w962) -> (index of element=w965:i32)  [unwired: 1 in]
                n562 = Equal?(x=w965, y=-1) -> (x = y?=w964:bool)
                n563 = case shown="True" w964 {
                  tunnel: w954 -> [w974 w988]
                  tunnel: w965 -> [w971 _]
                  tunnel: [w970 w987] -> w963
                  tunnel: w953 -> [_ w990]
                  tunnel: w962 -> [_ w977]
                  frame False {
                    n564 = local read "New: Temp"() -> (w968:dbl)
                    n565 = Divide(x=w971, y=3) -> (x/y=w973:dbl)
                    n566 = Format Value(format string="%#g", value (0)=w968) -> (output string=w967:string)  [unwired: 1 in]
                    n567 = To Word Integer(number=w973) -> (16bit integer=w972:i16)
                    n568 = Replace Array Subset(array=w974, new element=w967, index (row)=w972, index (col)=1) -> (w970:string[][])
                  }
                  frame True {
                    n569 = local read "New: Temp"() -> (w979:dbl)
                    n570 = Search 1D Array(1D array=w990, element="Width (um):") -> (index of element=w984:i32)  [unwired: 1 in]
                    n571 = Divide(x=w984, y=3) -> (x/y=w985:dbl)
                    n572 = To Word Integer(number=w985) -> (16bit integer=w983:i16)
                    n573 = Format Value(format string="%#g", value (0)=w979) -> (output string=w978:string)  [unwired: 1 in]
                    n574 = Build Array(w977, w978) -> (w981:string[])
                    n575 = Increment(x=w983) -> (x+1=w982:i16)
                    n576 = Insert Into Array(array=w988, index (row)=w982, new element=w981) -> (w987:string[][])  [unwired: 1 in]
                  }
                }
                n577 = local write "Save Array"(w963) -> ()
              }
              frame #5 {
                w1000 = "Mobility-Sat (cm^2/Vs):"
                n578 = local read "Save Array"() -> (w992:string[][])
                n579 = Array Size(array=w992) -> (size(s)=w997:i32[])
                n580 = Array Subset(array=w992, index (row)=0, index (col)=0, length (col)=3) -> (w993:string[][])  [unwired: 1 in]
                n581 = Index Array(array=w997, index=0) -> (element=w999:i32)
                n582 = Reshape Array(w993, w999) -> (w991:string[])
                n583 = Search 1D Array(1D array=w991, element=w1000) -> (index of element=w1003:i32)  [unwired: 1 in]
                n584 = Equal?(x=w1003, y=-1) -> (x = y?=w1002:bool)
                n585 = case shown="True" w1002 {
                  tunnel: w992 -> [w1013 w1023]
                  tunnel: w1003 -> [w1010 _]
                  tunnel: [w1009 w1022] -> w1001
                  tunnel: w991 -> [_ w1020]
                  tunnel: w1000 -> [_ w1018]
                  frame False {
                    n586 = local read "Re-Calculated Values Cluster"() -> (w1006:T10)
                    n587 = Unbundle By Name(w1006) -> ("Mobility-Sat"=w1005:dbl)
                    n588 = Divide(x=w1010, y=3) -> (x/y=w1012:dbl)
                    n589 = To Word Integer(number=w1012) -> (16bit integer=w1011:i16)
                    n590 = Format Value(format string="%#g", value (0)=w1005) -> (output string=w1007:string)  [unwired: 1 in]
                    n591 = Replace Array Subset(array=w1013, new element=w1007, index (row)=w1011, index (col)=1) -> (w1009:string[][])
                  }
                  frame True {
                    n592 = local read "Re-Calculated Values Cluster"() -> (w1017:T10)
                    n593 = Unbundle By Name(w1017) -> ("Mobility-Sat"=w1016:dbl)
                    n594 = Search 1D Array(1D array=w1020, element="Mobility (cm^2/Vs):") -> (index of element=w1026:i32)  [unwired: 1 in]
                    n595 = Divide(x=w1026, y=3) -> (x/y=w1027:dbl)
                    n596 = To Word Integer(number=w1027) -> (16bit integer=w1019:i16)
                    n597 = Format Value(format string="%#g", value (0)=w1016) -> (output string=w1021:string)  [unwired: 1 in]
                    n598 = Build Array(w1018, w1021) -> (w1025:string[])
                    n599 = Replace Array Subset(array=w1023, new element=w1025, index (row)=w1019) -> (w1022:string[][])  [unwired: 1 in]
                  }
                }
                n600 = local write "Save Array"(w1001) -> ()
              }
              frame #6 {
                w1039 = "Mobility-Lin (cm^2/Vs):"
                n601 = local read "Save Array"() -> (w1030:string[][])
                n602 = Array Size(array=w1030) -> (size(s)=w1036:i32[])
                n603 = Array Subset(array=w1030, index (row)=0, index (col)=0, length (col)=3) -> (w1032:string[][])  [unwired: 1 in]
                n604 = Index Array(array=w1036, index=0) -> (element=w1038:i32)
                n605 = Reshape Array(w1032, w1038) -> (w1031:string[])
                n606 = Search 1D Array(1D array=w1031, element=w1039) -> (index of element=w1042:i32)  [unwired: 1 in]
                n607 = Equal?(x=w1042, y=-1) -> (x = y?=w1041:bool)
                n608 = case shown="True" w1041 {
                  tunnel: w1030 -> [w1052 w1060]
                  tunnel: w1042 -> [w1049 _]
                  tunnel: [w1048 w1059] -> w1040
                  tunnel: w1031 -> [_ w1058]
                  tunnel: w1039 -> [_ w1057]
                  frame False {
                    n609 = local read "Re-Calculated Values Cluster"() -> (w1045:T10)
                    n610 = Unbundle By Name(w1045) -> ("Moblitity-Lin"=w1044:dbl)
                    n611 = Divide(x=w1049, y=3) -> (x/y=w1051:dbl)
                    n612 = To Word Integer(number=w1051) -> (16bit integer=w1050:i16)
                    n613 = Format Value(format string="%#g", value (0)=w1044) -> (output string=w1046:string)  [unwired: 1 in]
                    n614 = Replace Array Subset(array=w1052, new element=w1046, index (row)=w1050, index (col)=1) -> (w1048:string[][])
                  }
                  frame True {
                    n615 = local read "Re-Calculated Values Cluster"() -> (w1056:T10)
                    n616 = Unbundle By Name(w1056) -> ("Moblitity-Lin"=w1055:dbl)
                    n617 = Search 1D Array(1D array=w1058, element="Mobility-Sat (cm^2/Vs):") -> (index of element=w1065:i32)  [unwired: 1 in]
                    n618 = Divide(x=w1065, y=3) -> (x/y=w1066:dbl)
                    n619 = To Word Integer(number=w1066) -> (16bit integer=w1064:i16)
                    n620 = Format Value(format string="%#g", value (0)=w1055) -> (output string=w1069:string)  [unwired: 1 in]
                    n621 = Build Array(w1057, w1069) -> (w1062:string[])
                    n622 = Increment(x=w1064) -> (x+1=w1063:i16)
                    n623 = Insert Into Array(array=w1060, index (row)=w1063, new element=w1062) -> (w1059:string[][])  [unwired: 1 in]
                  }
                }
                n624 = local write "Save Array"(w1040) -> ()
              }
              frame #7 {
                w1079 = "On/Off I-Sat:"
                n625 = local read "Save Array"() -> (w1070:string[][])
                n626 = Array Size(array=w1070) -> (size(s)=w1076:i32[])
                n627 = Array Subset(array=w1070, index (row)=0, index (col)=0, length (col)=3) -> (w1072:string[][])  [unwired: 1 in]
                n628 = Index Array(array=w1076, index=0) -> (element=w1078:i32)
                n629 = Reshape Array(w1072, w1078) -> (w1071:string[])
                n630 = Search 1D Array(1D array=w1071, element=w1079) -> (index of element=w1082:i32)  [unwired: 1 in]
                n631 = Equal?(x=w1082, y=-1) -> (x = y?=w1081:bool)
                n632 = case shown="True" w1081 {
                  tunnel: w1070 -> [w1092 w1101]
                  tunnel: w1082 -> [w1089 _]
                  tunnel: [w1088 w1102] -> w1080
                  tunnel: w1071 -> [_ w1099]
                  tunnel: w1079 -> [_ w1097]
                  frame False {
                    n633 = local read "Calculated Values Cluster"() -> (w1085:T10)
                    n634 = Divide(x=w1089, y=3) -> (x/y=w1091:dbl)
                    n635 = Unbundle By Name(w1085) -> ("On/Off"=w1084:dbl)
                    n636 = To Word Integer(number=w1091) -> (16bit integer=w1090:i16)
                    n637 = Format Value(format string="%#g", value (0)=w1084) -> (output string=w1086:string)  [unwired: 1 in]
                    n638 = Replace Array Subset(array=w1092, new element=w1086, index (row)=w1090, index (col)=1) -> (w1088:string[][])
                  }
                  frame True {
                    n639 = local read "Calculated Values Cluster"() -> (w1096:T10)
                    n640 = Unbundle By Name(w1096) -> ("On/Off"=w1095:dbl)
                    n641 = Search 1D Array(1D array=w1099, element="On/Off Current:") -> (index of element=w1105:i32)  [unwired: 1 in]
                    n642 = Divide(x=w1105, y=3) -> (x/y=w1106:dbl)
                    n643 = To Word Integer(number=w1106) -> (16bit integer=w1098:i16)
                    n644 = Format Value(format string="%#g", value (0)=w1095) -> (output string=w1100:string)  [unwired: 1 in]
                    n645 = Build Array(w1097, w1100) -> (w1104:string[])
                    n646 = Replace Array Subset(array=w1101, new element=w1104, index (row)=w1098) -> (w1102:string[][])  [unwired: 1 in]
                  }
                }
                n647 = local write "Save Array"(w1080) -> ()
              }
              frame #8 {
                w1118 = "Off I-Sat (A):"
                n648 = local read "Save Array"() -> (w1109:string[][])
                n649 = Array Size(array=w1109) -> (size(s)=w1115:i32[])
                n650 = Array Subset(array=w1109, index (row)=0, index (col)=0, length (col)=3) -> (w1111:string[][])  [unwired: 1 in]
                n651 = Index Array(array=w1115, index=0) -> (element=w1117:i32)
                n652 = Reshape Array(w1111, w1117) -> (w1110:string[])
                n653 = Search 1D Array(1D array=w1110, element=w1118) -> (index of element=w1121:i32)  [unwired: 1 in]
                n654 = Equal?(x=w1121, y=-1) -> (x = y?=w1120:bool)
                n655 = case shown="True" w1120 {
                  tunnel: w1109 -> [w1131 w1139]
                  tunnel: w1121 -> [w1128 _]
                  tunnel: [w1127 w1138] -> w1119
                  tunnel: w1110 -> [_ w1137]
                  tunnel: w1118 -> [_ w1136]
                  frame False {
                    # "New Data File"
                    n656 = local read "Calculated Values Cluster"() -> (w1124:T10)
                    n657 = Unbundle By Name(w1124) -> ("Off Current"=w1123:dbl)
                    n658 = Divide(x=w1128, y=3) -> (x/y=w1130:dbl)
                    n659 = Format Value(format string="%#g", value (0)=w1123) -> (output string=w1125:string)  [unwired: 1 in]
                    n660 = To Word Integer(number=w1130) -> (16bit integer=w1129:i16)
                    n661 = Replace Array Subset(array=w1131, new element=w1125, index (row)=w1129, index (col)=1) -> (w1127:string[][])
                  }
                  frame True {
                    # "Old Data File"
                    n662 = local read "Calculated Values Cluster"() -> (w1135:T10)
                    n663 = Unbundle By Name(w1135) -> ("Off Current"=w1134:dbl)
                    n664 = Search 1D Array(1D array=w1137, element="On/Off I-Sat:") -> (index of element=w1144:i32)  [unwired: 1 in]
                    n665 = Divide(x=w1144, y=3) -> (x/y=w1145:dbl)
                    n666 = To Word Integer(number=w1145) -> (16bit integer=w1143:i16)
                    n667 = Format Value(format string="%#g", value (0)=w1134) -> (output string=w1148:string)  [unwired: 1 in]
                    n668 = Build Array(w1136, w1148) -> (w1141:string[])
                    n669 = Increment(x=w1143) -> (x+1=w1142:i16)
                    n670 = Insert Into Array(array=w1139, index (row)=w1142, new element=w1141) -> (w1138:string[][])  [unwired: 1 in]
                  }
                }
                n671 = local write "Save Array"(w1119) -> ()
              }
              frame #9 {
                w1150 = "Vt-Sat (V):"
                n672 = local read "Save Array"() -> (w1151:string[][])
                n673 = Array Size(array=w1151) -> (size(s)=w1156:i32[])
                n674 = Array Subset(array=w1151, index (row)=0, index (col)=0, length (col)=3) -> (w1152:string[][])  [unwired: 1 in]
                n675 = Index Array(array=w1156, index=0) -> (element=w1158:i32)
                n676 = Reshape Array(w1152, w1158) -> (w1149:string[])
                n677 = Search 1D Array(1D array=w1149, element=w1150) -> (index of element=w1161:i32)  [unwired: 1 in]
                n678 = Equal?(x=w1161, y=-1) -> (x = y?=w1160:bool)
                n679 = case shown="True" w1160 {
                  tunnel: w1151 -> [w1170 w1180]
                  tunnel: w1161 -> [w1166 _]
                  tunnel: [w1165 w1179] -> w1159
                  tunnel: w1150 -> [_ w1178]
                  tunnel: w1149 -> [_ w1177]
                  frame False {
                    n680 = local read "Re-Calculated Values Cluster"() -> (w1164:T10)
                    n681 = Unbundle By Name(w1164) -> ("Vt-Sat"=w1163:dbl)
                    n682 = Divide(x=w1166, y=3) -> (x/y=w1169:dbl)
                    n683 = To Word Integer(number=w1169) -> (16bit integer=w1168:i16)
                    n684 = Number To Fractional String(number=w1163) -> (F-format string=w1167:string)  [unwired: 3 in]
                    n685 = Replace Array Subset(array=w1170, new element=w1167, index (row)=w1168, index (col)=1) -> (w1165:string[][])
                  }
                  frame True {
                    n686 = local read "Re-Calculated Values Cluster"() -> (w1174:T10)
                    n687 = Unbundle By Name(w1174) -> ("Vt-Sat"=w1173:dbl)
                    n688 = Search 1D Array(1D array=w1177, element="Threshold V (V):") -> (index of element=w1176:i32)  [unwired: 1 in]
                    n689 = Divide(x=w1176, y=3) -> (x/y=w1183:dbl)
                    n690 = To Word Integer(number=w1183) -> (16bit integer=w1175:i16)
                    n691 = Format Value(format string="%#g", value (0)=w1173) -> (output string=w1186:string)  [unwired: 1 in]
                    n692 = Build Array(w1178, w1186) -> (w1182:string[])
                    n693 = Replace Array Subset(array=w1180, new element=w1182, index (row)=w1175) -> (w1179:string[][])  [unwired: 1 in]
                  }
                }
                n694 = local write "Save Array"(w1159) -> ()
              }
              frame #10 {
                n695 = disable-structure shown="Disabled" {
                  frame Disabled {
                    n696 = local read "Save Array"() -> (w1187:string[][])
                    n697 = Array Size(array=w1187) -> (size(s)=w1193:i32[])
                    n698 = Array Subset(array=w1187, index (row)=0, index (col)=0, length (col)=3) -> (w1189:string[][])  [unwired: 1 in]
                    n699 = Index Array(array=w1193, index=0) -> (element=w1195:i32)
                    n700 = Reshape Array(w1189, w1195) -> (w1188:string[])
                    n701 = Search 1D Array(1D array=w1188, element="VT-Lin (V):") -> (index of element=w1198:i32)  [unwired: 1 in]
                    n702 = Equal?(x=w1198, y=-1) -> (x = y?=w1197:bool)
                    n703 = case shown="False" w1197 {
                      tunnel: w1187 -> [w1207 w1210]
                      tunnel: w1198 -> [w1204 _]
                      tunnel: [w1203 w1210] -> w1196
                      frame False {
                        n704 = Divide(x=w1204, y=3) -> (x/y=w1206:dbl)
                        n705 = To Word Integer(number=w1206) -> (16bit integer=w1205:i16)
                        n706 = Format Value(format string="%#g") -> (output string=w1201:string)  [unwired: 2 in]
                        n707 = Replace Array Subset(array=w1207, new element=w1201, index (row)=w1205, index (col)=1) -> (w1203:string[][])
                      }
                      frame True {
                      }
                    }
                    n708 = local write "Save Array"(w1196) -> ()
                  }
                  frame Enabled {
                  }
                }
              }
              frame #11 {
                w1211 = "STS-Sat (V/decade):"
                n709 = local read "Save Array"() -> (w1213:string[][])
                n710 = Array Size(array=w1213) -> (size(s)=w1218:i32[])
                n711 = Array Subset(array=w1213, index (row)=0, index (col)=0, length (col)=3) -> (w1214:string[][])  [unwired: 1 in]
                n712 = Index Array(array=w1218, index=0) -> (element=w1220:i32)
                n713 = Reshape Array(w1214, w1220) -> (w1212:string[])
                n714 = Search 1D Array(1D array=w1212, element=w1211) -> (index of element=w1223:i32)  [unwired: 1 in]
                n715 = Equal?(x=w1223, y=-1) -> (x = y?=w1222:bool)
                n716 = case shown="True" w1222 {
                  tunnel: w1213 -> [w1233 w1241]
                  tunnel: w1223 -> [w1230 _]
                  tunnel: [w1229 w1242] -> w1221
                  tunnel: w1212 -> [_ w1240]
                  tunnel: w1211 -> [_ w1239]
                  frame False {
                    # "Current Data File"
                    n717 = local read "Re-Calculated Values Cluster"() -> (w1225:T10)
                    n718 = Unbundle By Name(w1225) -> ("STS"=w1226:dbl)
                    n719 = Divide(x=w1230, y=3) -> (x/y=w1232:dbl)
                    n720 = To Word Integer(number=w1232) -> (16bit integer=w1231:i16)
                    n721 = Format Value(format string="%#g", value (0)=w1226) -> (output string=w1227:string)  [unwired: 1 in]
                    n722 = Replace Array Subset(array=w1233, new element=w1227, index (row)=w1231, index (col)=1) -> (w1229:string[][])
                  }
                  frame True {
                    # "Old Data File"
                    n723 = local read "Re-Calculated Values Cluster"() -> (w1236:T10)
                    n724 = Unbundle By Name(w1236) -> ("STS"=w1237:dbl)
                    n725 = Search 1D Array(1D array=w1240, element="S.T.S. (V/decade):") -> (index of element=w1245:i32)  [unwired: 1 in]
                    n726 = Divide(x=w1245, y=3) -> (x/y=w1246:dbl)
                    n727 = To Word Integer(number=w1246) -> (16bit integer=w1238:i16)
                    n728 = Format Value(format string="%#g", value (0)=w1237) -> (output string=w1249:string)  [unwired: 1 in]
                    n729 = Build Array(w1239, w1249) -> (w1244:string[])
                    n730 = Replace Array Subset(array=w1241, new element=w1244, index (row)=w1238) -> (w1242:string[][])  [unwired: 1 in]
                  }
                }
                n731 = local write "Save Array"(w1221) -> ()
              }
              frame #12 {
                w1250 = "Trap Density-VT (Traps/Vcm^2):"
                n732 = local read "Save Array"() -> (w1252:string[][])
                n733 = Array Size(array=w1252) -> (size(s)=w1257:i32[])
                n734 = Array Subset(array=w1252, index (row)=0, index (col)=0, length (col)=3) -> (w1253:string[][])  [unwired: 1 in]
                n735 = Index Array(array=w1257, index=0) -> (element=w1259:i32)
                n736 = Reshape Array(w1253, w1259) -> (w1251:string[])
                n737 = Search 1D Array(1D array=w1251, element=w1250) -> (index of element=w1262:i32)  [unwired: 1 in]
                n738 = Equal?(x=w1262, y=-1) -> (x = y?=w1261:bool)
                n739 = case shown="True" w1261 {
                  tunnel: w1252 -> [w1272 w1279]
                  tunnel: w1262 -> [w1268 _]
                  tunnel: [w1267 w1280] -> w1260
                  tunnel: w1251 -> [_ w1278]
                  tunnel: w1250 -> [_ w1277]
                  frame False {
                    n740 = local read "Re-Calculated Values Cluster"() -> (w1265:T10)
                    n741 = Unbundle By Name(w1265) -> ("Trap Density-VT"=w1264:dbl)
                    n742 = Divide(x=w1268, y=3) -> (x/y=w1271:dbl)
                    n743 = To Word Integer(number=w1271) -> (16bit integer=w1270:i16)
                    n744 = Format Value(format string="%#g", value (0)=w1264) -> (output string=w1269:string)  [unwired: 1 in]
                    n745 = Replace Array Subset(array=w1272, new element=w1269, index (row)=w1270, index (col)=1) -> (w1267:string[][])
                  }
                  frame True {
                    n746 = local read "Re-Calculated Values Cluster"() -> (w1276:T10)
                    n747 = Unbundle By Name(w1276) -> ("Trap Density-VT"=w1275:dbl)
                    n748 = Search 1D Array(1D array=w1278, element="STS-Sat (V/decade):") -> (index of element=w1285:i32)  [unwired: 1 in]
                    n749 = Divide(x=w1285, y=3) -> (x/y=w1284:dbl)
                    n750 = To Word Integer(number=w1284) -> (16bit integer=w1286:i16)
                    n751 = Format Value(format string="%#g", value (0)=w1275) -> (output string=w1281:string)  [unwired: 1 in]
                    n752 = Build Array(w1277, w1281) -> (w1288:string[])
                    n753 = Increment(x=w1286) -> (x+1=w1287:i16)
                    n754 = Insert Into Array(array=w1279, index (row)=w1287, new element=w1288) -> (w1280:string[][])  [unwired: 1 in]
                  }
                }
                n755 = local write "Save Array"(w1260) -> ()
              }
              frame #13 {
                w1290 = "Trap Density-STS (Traps/Vcm^2):"
                n756 = local read "Save Array"() -> (w1292:string[][])
                n757 = Array Size(array=w1292) -> (size(s)=w1297:i32[])
                n758 = Array Subset(array=w1292, index (row)=0, index (col)=0, length (col)=3) -> (w1293:string[][])  [unwired: 1 in]
                n759 = Index Array(array=w1297, index=0) -> (element=w1299:i32)
                n760 = Reshape Array(w1293, w1299) -> (w1291:string[])
                n761 = Search 1D Array(1D array=w1291, element=w1290) -> (index of element=w1302:i32)  [unwired: 1 in]
                n762 = Equal?(x=w1302, y=-1) -> (x = y?=w1301:bool)
                n763 = case shown="True" w1301 {
                  tunnel: w1292 -> [w1312 w1319]
                  tunnel: w1302 -> [w1309 _]
                  tunnel: [w1308 w1320] -> w1300
                  tunnel: w1291 -> [_ w1318]
                  tunnel: w1290 -> [_ w1317]
                  frame False {
                    n764 = local read "Re-Calculated Values Cluster"() -> (w1305:T10)
                    n765 = Unbundle By Name(w1305) -> ("Trap Density-STS"=w1304:dbl)
                    n766 = Divide(x=w1309, y=3) -> (x/y=w1311:dbl)
                    n767 = To Word Integer(number=w1311) -> (16bit integer=w1310:i16)
                    n768 = Format Value(format string="%#g", value (0)=w1304) -> (output string=w1306:string)  [unwired: 1 in]
                    n769 = Replace Array Subset(array=w1312, new element=w1306, index (row)=w1310, index (col)=1) -> (w1308:string[][])
                  }
                  frame True {
                    n770 = local read "Re-Calculated Values Cluster"() -> (w1316:T10)
                    n771 = Unbundle By Name(w1316) -> ("Trap Density-STS"=w1315:dbl)
                    n772 = Search 1D Array(1D array=w1318, element="Trap Density-VT (Traps/Vcm^2):") -> (index of element=w1325:i32)  [unwired: 1 in]
                    n773 = Divide(x=w1325, y=3) -> (x/y=w1326:dbl)
                    n774 = To Word Integer(number=w1326) -> (16bit integer=w1324:i16)
                    n775 = Format Value(format string="%#g", value (0)=w1315) -> (output string=w1329:string)  [unwired: 1 in]
                    n776 = Build Array(w1317, w1329) -> (w1322:string[])
                    n777 = Increment(x=w1324) -> (x+1=w1323:i16)
                    n778 = Insert Into Array(array=w1319, index (row)=w1323, new element=w1322) -> (w1320:string[][])  [unwired: 1 in]
                  }
                }
                n779 = local write "Save Array"(w1300) -> ()
              }
            }
            n780 = local read "New: Temp"() -> (w837:dbl)
            n781 = local read "New: Width"() -> (w838:dbl)
            n782 = local read "New: Length"() -> (w840:dbl)
            n783 = local read "Index"() -> (w839:string)
            n784 = To Single Precision Float(number=w837) -> (single precision float=w854:sgl)
            n785 = Number To Decimal String(number=w854) -> (decimal integer string=w849:string)  [unwired: 1 in]
            n786 = To Single Precision Float(number=w838) -> (single precision float=w853:sgl)
            n787 = To Single Precision Float(number=w840) -> (single precision float=w852:sgl)
            n788 = Strip Path(path=w836) -> (stripped path=w841:path)  [unwired: 1 out]
            n789 = Number To Decimal String(number=w852) -> (decimal integer string=w847:string)  [unwired: 1 in]
            n790 = Number To Decimal String(number=w853) -> (decimal integer string=w846:string)  [unwired: 1 in]
            n791 = Concatenate Strings("_", w849, "K") -> (w851:string)
            n792 = call "Build Text"("Temp"=w851, "Index"=w839, "Length"=w847, "Width"=w846) -> ("Result"=w845:string)  [unwired: 10 in, 1 out]
            n793 = Path To String(path=w841) -> (string=w843:string)
            n794 = Concatenate Strings(w843, "\\", w845) -> (w844:string)
            n795 = String To Path(string=w844) -> (path=w835:path)
          }
          frame #1 {
            n796 = flat-sequence {
              tunnel: w1333 -> [w1335]
              tunnel: w1332 -> [w1334]
              tunnel: [w1334] -> w1331
              tunnel: w1331 -> [w1341]
              tunnel: w1330 -> [w1340]
              frame #0 {
                n797 = Equal?(x=w1335, y=w1334) -> (x = y?=w1336:bool)
                n798 = case shown="False" w1336 {
                  tunnel: w1335 -> [w1339 _]
                  tunnel: w1334 -> [w1338 _]
                  frame False {
                    n799 = Move(source path=w1339, 9:TRUE, 10:w1338) -> ()  [unwired: 2 in, 3 out]
                  }
                  frame True {
                  }
                }
              }
              frame #1 {
                n800 = local write "Transfer File"(w1341) -> ()
                n801 = call-poly <vilib>:"Write To Spreadsheet File.vi"("2D data"=w1340, "file path (dialog if empty)"=w1341) -> ()  [unwired: 6 in, 1 out]
              }
            }
          }
        }
        n802 = Unbundle By Name(w821) -> ("Save Next"=w820:bool)
        n803 = Cluster To Array(cluster=w826) -> (array=w825:bool[])
        n804 = Boolean Array To Number(Boolean array=w825) -> (number=w824:u32)
        n805 = Equal To 0?(x=w824) -> (x = 0?=w823:bool)
        n806 = case shown="True" w823 {
          tunnel: [MegaAwesome_States."Read Data" w833] -> w822
          tunnel: w820 -> [_ w830]
          frame False {
          }
          frame True {
            n807 = Select(t=MegaAwesome_States."No Event", s=w830, f=MegaAwesome_States."Next File") -> (s? t:f=w833:T3)
          }
        }
      }
      frame "Exit" {
        n808 = call "IMAQ Dispose"("All Images? (No)"=TRUE) -> ()  [unwired: 5 in, 1 out]
      }
      frame "Save Lines" {
        n809 = Build Path(base path=w1346, name or relative path="ROI") -> (appended path=w1349:path)
        n810 = call <vilib>:"Check if File or Folder Exists.vi"("path"=w1349) -> ("file or folder exists?"=w1347:bool, "dup path"=w1350:path)  [unwired: 8 in, 1 out]
        n811 = case shown="False" w1347 {
          tunnel: w1350 -> [w1358 w1359]
          tunnel: [w1357 w1359] -> w1354
          frame False {
            n812 = Create Folder(path (use dialog)=w1358) -> (created path=w1357:path)  [unwired: 2 in, 2 out]
          }
          frame True {
          }
        }
        n813 = local read "Index"() -> (w1345:string)
        n814 = property on="Image Out" class="ImageControl"() -> ("ROI"=w1351:T13)  [unwired: 2 in, 2 out]
        n815 = Build Path(base path=w1354, name or relative path=w1345) -> (appended path=w1353:path)
        n816 = Flatten To String(anything=w1351) -> (data string=w1352:string)  [unwired: 3 in, 2 out]
        n817 = Write to Text File(file (use dialog)=w1353, text=w1352) -> ()  [unwired: 2 in, 3 out]
      }
      frame "Export" {
        n818 = flat-sequence {
          tunnel: w1360 -> [w1413]
          frame #0 {
            n819 = stacked-sequence {
              frame #0 {
                n820 = local read "Independant Variable:"() -> (w1363:string)
                n821 = Equal?(x=w1363, y="Length (um):") -> (x = y?=w1364:bool)
                n822 = case shown="True" w1364 {
                  frame False {
                  }
                  frame True {
                    n823 = local write "X Axis Display Type"("1") -> ()
                    n824 = local write "Opj X Axis"("2") -> ()
                  }
                }
              }
              frame #1 {
                n825 = local read "Independant Variable:"() -> (w1368:string)
                n826 = Equal?(x=w1368, y="Sample Temp (K):") -> (x = y?=w1369:bool)
                n827 = case shown="True" w1369 {
                  frame False {
                  }
                  frame True {
                    n828 = local write "X Axis Display Type"("1") -> ()
                    n829 = local write "Opj X Axis"("1") -> ()
                  }
                }
              }
              frame #2 {
                n830 = local read "Independant Variable:"() -> (w1373:string)
                n831 = Equal?(x=w1373, y="Mobility-Sat (cm^2/Vs):") -> (x = y?=w1374:bool)
                n832 = case shown="True" w1374 {
                  frame False {
                  }
                  frame True {
                    n833 = local write "X Axis Display Type"("2") -> ()
                    n834 = local write "Opj X Axis"("2") -> ()
                  }
                }
              }
              frame #3 {
                n835 = local read "Independant Variable:"() -> (w1378:string)
                n836 = Equal?(x=w1378, y="Mobility-Lin (cm^2/Vs):") -> (x = y?=w1379:bool)
                n837 = case shown="True" w1379 {
                  frame False {
                  }
                  frame True {
                    n838 = local write "X Axis Display Type"("2") -> ()
                    n839 = local write "Opj X Axis"("2") -> ()
                  }
                }
              }
              frame #4 {
                n840 = local read "Independant Variable:"() -> (w1383:string)
                n841 = Equal?(x=w1383, y="On/Off I-Sat:") -> (x = y?=w1384:bool)
                n842 = case shown="True" w1384 {
                  frame False {
                  }
                  frame True {
                    n843 = local write "X Axis Display Type"("2") -> ()
                    n844 = local write "Opj X Axis"("2") -> ()
                  }
                }
              }
              frame #5 {
                n845 = local read "Independant Variable:"() -> (w1388:string)
                n846 = Equal?(x=w1388, y="Off I-Sat (A):") -> (x = y?=w1389:bool)
                n847 = case shown="True" w1389 {
                  frame False {
                  }
                  frame True {
                    n848 = local write "X Axis Display Type"("2") -> ()
                    n849 = local write "Opj X Axis"("2") -> ()
                  }
                }
              }
              frame #6 {
                n850 = local read "Independant Variable:"() -> (w1393:string)
                n851 = Equal?(x=w1393, y="Vt-Sat (V):") -> (x = y?=w1394:bool)
                n852 = case shown="True" w1394 {
                  frame False {
                  }
                  frame True {
                    n853 = local write "X Axis Display Type"("1") -> ()
                    n854 = local write "Opj X Axis"("1") -> ()
                  }
                }
              }
              frame #7 {
                n855 = local read "Independant Variable:"() -> (w1398:string)
                n856 = Equal?(x=w1398, y="STS-Sat (V/decade):") -> (x = y?=w1399:bool)
                n857 = case shown="True" w1399 {
                  frame False {
                  }
                  frame True {
                    n858 = local write "X Axis Display Type"("1") -> ()
                    n859 = local write "Opj X Axis"("1") -> ()
                  }
                }
              }
              frame #8 {
                n860 = local read "Independant Variable:"() -> (w1403:string)
                n861 = Equal?(x=w1403, y="Trap Density-VT (Traps/Vcm^2):") -> (x = y?=w1404:bool)
                n862 = case shown="True" w1404 {
                  frame False {
                  }
                  frame True {
                    n863 = local write "X Axis Display Type"("2") -> ()
                    n864 = local write "Opj X Axis"("2") -> ()
                  }
                }
              }
              frame #9 {
                n865 = local read "Independant Variable:"() -> (w1408:string)
                n866 = Equal?(x=w1408, y="Trap Density-STS (Traps/Vcm^2):") -> (x = y?=w1409:bool)
                n867 = case shown="True" w1409 {
                  frame False {
                  }
                  frame True {
                    n868 = local write "X Axis Display Type"("2") -> ()
                    n869 = local write "Opj X Axis"("2") -> ()
                  }
                }
              }
            }
          }
          frame #1 {
            n870 = local read "Transfer Folder"() -> (w1418:path)
            n871 = Build Path(base path=w1418, name or relative path="Stats") -> (appended path=w1419:path)
            n872 = call <vilib>:"Check if File or Folder Exists.vi"("path"=w1419) -> ("file or folder exists?"=w1433:bool, "dup path"=w1432:path)  [unwired: 8 in, 1 out]
            n873 = call <userlib>:"OA_ConnectToOrigin.vi"() -> ("error out"=w1430:errorcluster, "Origin.IOApplication"=w1431:refnum<k7>)  [unwired: 8 in]
            n874 = case shown="False" w1433 {
              tunnel: w1432 -> [w1606 w1607]
              tunnel: [w1605 w1607] -> w1417
              frame False {
                n875 = Create Folder(path (use dialog)=w1606) -> (created path=w1605:path)  [unwired: 2 in, 2 out]
              }
              frame True {
              }
            }
            n876 = call "File Dialog"("start path"=w1419) -> ("selected path"=w1421:path)  [unwired: 11 in, 3 out]
            n877 = call <userlib>:"OA_Load.vi"("error in (no error)"=w1430, "Path"=w1413, "Origin.IOApplication"=w1431) -> ("error out"=w1428:errorcluster, "Origin.IOApplication"=w1429:refnum<k7>)  [unwired: 1 out]
            n878 = call "OAExecute.vi"("script"="document -m 3;", "Error IO"=w1428, "Origin.IOApplication"=w1429) -> ("Error IO Out"=w1426:errorcluster, "Origin.IOApplication"=w1427:refnum<k7>)  [unwired: 1 in, 1 out]
            n879 = local read "Independant Variable:"() -> (w1414:string)
            n880 = stacked-sequence {
              tunnel: w1418 -> [w1444 w1474 w1486 w1508 w1528 w1549 w1570 w1593]
              tunnel: w1417 -> [w1445 w1473 w1487 w1507 w1529 w1550 w1571 w1594]
              tunnel: w1427 -> [w1447 w1471 w1489 w1510 w1531 w1552 w1573 w1596]
              tunnel: w1426 -> [w1446 w1472 w1488 w1509 w1530 w1551 w1572 w1595]
              tunnel: [_ _ _ _ _ _ _ w1591] -> w1416
              tunnel: [_ _ _ _ _ _ _ w1592] -> w1415
              tunnel: w1414 -> [w1443 w1464 w1485 w1506 w1527 w1548 w1569 w1590]
              frame #0 {
                n881 = local read "X Axis Display Type"() -> (w1435:string)
                n882 = local read "Opj X Axis"() -> (w1440:string)
                n883 = Concatenate Strings("window -a MOBLGraph;\nlayer.x.type=", w1440, "; layer.x.label.numFormat = ", w1435, "; Y3 = 1; X3 = 1;", "window -a MOBLTable;\nwindow -s TV;") -> (w1438:string)
                n884 = call "Param_Analysis_7_24b_JW.vi"("Independant Variable"=w1443, "error in (no error)"=w1446, "Data Folder"=w1444, "Parameter String"="Mobility-Lin (cm^2/Vs):", "Parameter Name"="Mobility-Lin", "Stats Folder"=w1445) -> ("error out"=w1449:errorcluster, "Output Array"=w1451:string[][], "Variables"=w1442:T27)  [unwired: 2 in, 1 out]
                n885 = call "Origin_Export_7_27a_JW.vi"("Input Conditions"=w1442, "Analysis Array"=w1451, "error in (no error)"=w1449, "Parameter Worksheet Name"="[MOBLTable]Mobilities", "Parameter Folder Script"="pe_cd \"Mobility-Lin\";", "Origin.IOApplication"=w1447) -> ("error out"=w1448:errorcluster, "reference out"=w1450:refnum<k7>)  [unwired: 3 in, 1 out]
                n886 = call "OAExecute.vi"("script"=w1438, "Error IO"=w1448, "Origin.IOApplication"=w1450) -> ()  [unwired: 1 in, 3 out]
              }
              frame #1 {
                n887 = local read "X Axis Display Type"() -> (w1456:string)
                n888 = local read "Opj X Axis"() -> (w1461:string)
                n889 = Concatenate Strings("window -a MOBSGraph;\nlayer.x.type=", w1461, "; layer.x.label.numFormat = ", w1456, "; Y3 = 1; X3 = 1;", "window -a MOBSTable;\nwindow -s TV;") -> (w1459:string)
                n890 = call "Param_Analysis_7_24b_JW.vi"("Independant Variable"=w1464, "error in (no error)"=w1472, "Data Folder"=w1474, "Parameter String"="Mobility-Sat (cm^2/Vs):", "Parameter Name"="Mobility-Sat", "Stats Folder"=w1473) -> ("error out"=w1467:errorcluster, "Output Array"=w1465:string[][], "Variables"=w1463:T27)  [unwired: 2 in, 1 out]
                n891 = call "Origin_Export_7_27a_JW.vi"("Input Conditions"=w1463, "Analysis Array"=w1465, "error in (no error)"=w1467, "Parameter Worksheet Name"="[MOBSTable]Mobilities", "Parameter Folder Script"="pe_cd \"Mobility-Sat\";", "Origin.IOApplication"=w1471) -> ("error out"=w1466:errorcluster, "reference out"=w1468:refnum<k7>)  [unwired: 3 in, 1 out]
                n892 = call "OAExecute.vi"("script"=w1459, "Error IO"=w1466, "Origin.IOApplication"=w1468) -> ()  [unwired: 1 in, 3 out]
              }
              frame #2 {
                n893 = local read "X Axis Display Type"() -> (w1477:string)
                n894 = local read "Opj X Axis"() -> (w1482:string)
                n895 = Concatenate Strings("window -a NSTSGraph;\nlayer.x.type=", w1482, "; layer.x.label.numFormat = ", w1477, "; Y3 = 1; X3 = 1;", "window -a NSTSTable;\nwindow -s TV;") -> (w1480:string)
                n896 = call "Param_Analysis_7_24b_JW.vi"("Independant Variable"=w1485, "error in (no error)"=w1488, "Data Folder"=w1486, "Parameter String"="Trap Density-STS (Traps/Vcm^2):", "Parameter Name"="Trap Density-STS", "Stats Folder"=w1487) -> ("error out"=w1492:errorcluster, "Output Array"=w1490:string[][], "Variables"=w1484:T27)  [unwired: 2 in, 1 out]
                n897 = call "Origin_Export_7_27a_JW.vi"("Input Conditions"=w1484, "Analysis Array"=w1490, "error in (no error)"=w1492, "Parameter Worksheet Name"="[NSTSTable]Trap Densities", "Parameter Folder Script"="pe_cd \"N-STS\";", "Origin.IOApplication"=w1489) -> ("error out"=w1491:errorcluster, "reference out"=w1493:refnum<k7>)  [unwired: 3 in, 1 out]
                n898 = call "OAExecute.vi"("script"=w1480, "Error IO"=w1491, "Origin.IOApplication"=w1493) -> ()  [unwired: 1 in, 3 out]
              }
              frame #3 {
                n899 = local read "X Axis Display Type"() -> (w1498:string)
                n900 = local read "Opj X Axis"() -> (w1503:string)
                n901 = call "Param_Analysis_7_24b_JW.vi"("Independant Variable"=w1506, "error in (no error)"=w1509, "Data Folder"=w1508, "Parameter String"="Trap Density-VT (Traps/Vcm^2):", "Parameter Name"="Trap Density-Vt", "Stats Folder"=w1507) -> ("error out"=w1513:errorcluster, "Output Array"=w1511:string[][], "Variables"=w1505:T27)  [unwired: 2 in, 1 out]
                n902 = Concatenate Strings("window -a NVtGraph;\nlayer.x.type=", w1503, "; layer.x.label.numFormat = ", w1498, "; Y3 = 1; X3 = 1;", "window -a NVtTable;\nwindow -s TV;") -> (w1501:string)
                n903 = call "Origin_Export_7_27a_JW.vi"("Input Conditions"=w1505, "Analysis Array"=w1511, "error in (no error)"=w1513, "Parameter Worksheet Name"="[NVTTable]Trap Densities", "Parameter Folder Script"="pe_cd \"N-Vt\";", "Origin.IOApplication"=w1510) -> ("error out"=w1512:errorcluster, "reference out"=w1514:refnum<k7>)  [unwired: 3 in, 1 out]
                n904 = call "OAExecute.vi"("script"=w1501, "Error IO"=w1512, "Origin.IOApplication"=w1514) -> ()  [unwired: 1 in, 3 out]
              }
              frame #4 {
                n905 = local read "X Axis Display Type"() -> (w1519:string)
                n906 = local read "Opj X Axis"() -> (w1524:string)
                n907 = Concatenate Strings("window -a OffIGraph;\nlayer.x.type=", w1524, "; layer.x.label.numFormat = ", w1519, "; Y3 = 1; X3 = 1;", "window -a OffITable;\nwindow -s TV;") -> (w1522:string)
                n908 = call "Param_Analysis_7_24b_JW.vi"("Independant Variable"=w1527, "error in (no error)"=w1530, "Data Folder"=w1528, "Parameter String"="Off I-Sat (A):", "Parameter Name"="Off I-Sat", "Stats Folder"=w1529) -> ("error out"=w1534:errorcluster, "Output Array"=w1532:string[][], "Variables"=w1526:T27)  [unwired: 2 in, 1 out]
                n909 = call "Origin_Export_7_27a_JW.vi"("Input Conditions"=w1526, "Analysis Array"=w1532, "error in (no error)"=w1534, "Parameter Worksheet Name"="[OffItable]OffCurrents", "Parameter Folder Script"="pe_cd \"OffI-Sat\";", "Origin.IOApplication"=w1531) -> ("error out"=w1533:errorcluster, "reference out"=w1535:refnum<k7>)  [unwired: 3 in, 1 out]
                n910 = call "OAExecute.vi"("script"=w1522, "Error IO"=w1533, "Origin.IOApplication"=w1535) -> ()  [unwired: 1 in, 3 out]
              }
              frame #5 {
                n911 = local read "X Axis Display Type"() -> (w1540:string)
                n912 = local read "Opj X Axis"() -> (w1545:string)
                n913 = Concatenate Strings("window -a OnOffGraph;\nlayer.x.type=", w1545, "; layer.x.label.numFormat = ", w1540, "; Y3 = 1; X3 = 1;", "window -a OnOffTable;\nwindow -s TV;") -> (w1543:string)
                n914 = call "Param_Analysis_7_24b_JW.vi"("Independant Variable"=w1548, "error in (no error)"=w1551, "Data Folder"=w1549, "Parameter String"="On/Off I-Sat:", "Parameter Name"="OnOff Ratio", "Stats Folder"=w1550) -> ("error out"=w1555:errorcluster, "Output Array"=w1553:string[][], "Variables"=w1547:T27)  [unwired: 2 in, 1 out]
                n915 = call "Origin_Export_7_27a_JW.vi"("Input Conditions"=w1547, "Analysis Array"=w1553, "error in (no error)"=w1555, "Parameter Worksheet Name"="[OnOffTable]On/Off Ratios", "Parameter Folder Script"="pe_cd \"OnOff-Ratio\";", "Origin.IOApplication"=w1552) -> ("error out"=w1554:errorcluster, "reference out"=w1556:refnum<k7>)  [unwired: 3 in, 1 out]
                n916 = call "OAExecute.vi"("script"=w1543, "Error IO"=w1554, "Origin.IOApplication"=w1556) -> ()  [unwired: 1 in, 3 out]
              }
              frame #6 {
                n917 = local read "X Axis Display Type"() -> (w1561:string)
                n918 = local read "Opj X Axis"() -> (w1566:string)
                n919 = call "Param_Analysis_7_24b_JW.vi"("Independant Variable"=w1569, "error in (no error)"=w1572, "Data Folder"=w1570, "Parameter String"="STS-Sat (V/decade):", "Parameter Name"="STS-Sat", "Stats Folder"=w1571) -> ("error out"=w1576:errorcluster, "Output Array"=w1574:string[][], "Variables"=w1568:T27)  [unwired: 2 in, 1 out]
                n920 = Concatenate Strings("window -a SGraph;\nlayer.x.type=", w1566, "; layer.x.label.numFormat = ", w1561, "; Y3 = 1; X3 = 1;", "window -a STable;\nwindow -s TV;") -> (w1564:string)
                n921 = call "Origin_Export_7_27a_JW.vi"("Input Conditions"=w1568, "Analysis Array"=w1574, "error in (no error)"=w1576, "Parameter Worksheet Name"="[STable]Threshold Swing", "Parameter Folder Script"="pe_cd \"STS-Sat\";", "Origin.IOApplication"=w1573) -> ("error out"=w1575:errorcluster, "reference out"=w1577:refnum<k7>)  [unwired: 3 in, 1 out]
                n922 = call "OAExecute.vi"("script"=w1564, "Error IO"=w1575, "Origin.IOApplication"=w1577) -> ()  [unwired: 1 in, 3 out]
              }
              frame #7 {
                n923 = local read "X Axis Display Type"() -> (w1582:string)
                n924 = local read "Opj X Axis"() -> (w1587:string)
                n925 = Concatenate Strings("window -a VtGraph;\nlayer.x.type=", w1587, "; layer.x.label.numFormat = ", w1582, "; Y3 = 1; X3 = 1;", "window -a VtTable;\nwindow -s TV;") -> (w1585:string)
                n926 = call "Param_Analysis_7_24b_JW.vi"("Independant Variable"=w1590, "error in (no error)"=w1595, "Data Folder"=w1593, "Parameter String"="Vt-Sat (V):", "Parameter Name"="Vt-Sat", "Stats Folder"=w1594) -> ("error out"=w1599:errorcluster, "Output Array"=w1597:string[][], "Variables"=w1589:T27)  [unwired: 2 in, 1 out]
                n927 = call "Origin_Export_7_27a_JW.vi"("Input Conditions"=w1589, "Analysis Array"=w1597, "error in (no error)"=w1599, "Parameter Worksheet Name"="[VtTable]Threshold Voltages", "Parameter Folder Script"="pe_cd \"Vt-Sat\";", "Origin.IOApplication"=w1596) -> ("error out"=w1598:errorcluster, "reference out"=w1600:refnum<k7>)  [unwired: 3 in, 1 out]
                n928 = call "OAExecute.vi"("script"=w1585, "Error IO"=w1598, "Origin.IOApplication"=w1600) -> ("Error IO Out"=w1591:errorcluster, "Origin.IOApplication"=w1592:refnum<k7>)  [unwired: 1 in, 1 out]
              }
            }
            n929 = Path To String(path=w1421) -> (string=w1420:string)
            n930 = call "OAExecute.vi"("script"="pe_cd /; ", "Error IO"=w1416, "Origin.IOApplication"=w1415) -> ("Error IO Out"=w1422:errorcluster, "Origin.IOApplication"=w1423:refnum<k7>)  [unwired: 1 in, 1 out]
            n931 = call <userlib>:"OASaveProject.vi"("path"=w1420, "Error IO"=w1422, "Origin.IOApplication"=w1423) -> ()  [unwired: 3 out]
          }
        }
      }
    }
    "Current State" <- w10
    "Folder Index" <- w22
    n932 = Wait (ms)(milliseconds to wait=w16) -> ()  [unwired: 1 out]
    n933 = Equal?(x=w10, y=MegaAwesome_States."Exit") -> (x = y?=w30:bool)
  }
